vi "GUI.vi"() -> ()   [LabVIEW 2021]
uses:
  controls/ID Selector.ctl
  controls/UI Data.ctl
  controls/Data.ctl
  controls/ID.ctl
  controls/TCP states.ctl
  059b9806-6a42-4b51-9632-7dd4716d5fea.vi
  d48d9fbf-083e-4a49-8357-be6f50655bb8.vi
  d1c76d09-55ba-46af-828f-de7639a0dcdd.vi
  95893427-e2d0-46a1-b4a3-4e70b98dcc16.vi
  2dad5fc2-64a7-4bc6-978c-59d02dfdd1f4.vi
  2949da81-479a-477f-9d10-411d5337d71f.vi
  442cc11d-0c4b-4e6f-9aab-44bad20e65cf.vi
  aef3fa8d-d4ae-4391-a8c5-cd918d9f83e5.vi
  a61ae134-ce90-4c24-9a04-42d570ae496f.vi
  f3131f72-7d98-4291-8b40-3e2eb76ee77d.vi
  86390890-2633-40e9-acce-cca27de463dd.vi
  2bda4b71-a642-41ec-971a-aac1149cdb2e.vi
  4ba25f78-e02b-4593-a0a9-e7bfe2c227aa.vi
  b19a6172-c0db-45aa-bd96-f9eb8b4476d0.vi
  58187356-d8b0-41a2-b154-68928c7ad215.vi
  a77830ea-4afa-4eae-8504-e764fa7f6393.vi
  64a5f718-e64e-4ef8-854d-0519ac11c647.vi
  a36a24be-52b4-40ff-a07c-4f3c681fa51a.vi
  a822a74e-ca46-421e-8eac-677a4dba8bc9.vi
  651c30db-6f4a-4395-b9ba-95e4c80eae7c.vi
  ebd5c18a-2623-4cb2-8f61-688916ea3a38.vi
  3a8d74db-b308-4837-9c6e-c7dbc4062129.vi
  <vilib>/Utility/error.llb/Error Cluster From Error Code.vi
  styles/colors.vi
  <vilib>/ErrorRing/Error Ring.xnode
panel:
  out "ID:":string
  in  "Open part #":bool
  out "Parte number":string
  in  "Mode label":string="Mode:"
  in  "Options Button":bool
  in  "Mode:":T1
  in  "Start Button":bool
  out "Tab Control":enum32{"Micros", "Micro", "SSH"}(tab)
  in  "DH":bool
  in  "WH":bool
  in  "DA":bool
  in  "WM":bool
  in  "WA":bool
  in  "WC":bool
  in  "DS":bool
  in  "WS":bool
  in  "DM":bool
  in  "DC":bool
  in  "SM":bool
  in  "PWR":bool
  out "WS":string
  out "DS":string
  out "DM":string
  out "DC":string
  out "SM":string
  out "PWR":string
  out "WH":string
  out "DH":string
  out "DA":string
  out "WM":string
  out "WA":string
  out "WC":string
  out "Pass or fail":string
  out "Status":string caption="Conexión TCP-IP"
  out "version:":string
  in  "Save Button":bool
  in  "Path: 4.9.12.XXXX":path=path "C:/Users/ken_X/Documents/LabVIEW projects/Project-A/outset-medical/4.9.12.6034"
  in  "Path: Mi app":path=path "C:/Users/ken_X/Documents/LabVIEW projects/Project-A/outset-medical/Android OS"
  # "WS"
  # "DS"
  # "PWR"
  # "DM"
  # "SM"
  # "DC"
  # "WC"
  # "WH"
  # "DH"
  # "DA"
  # "WA"
  # "WM"
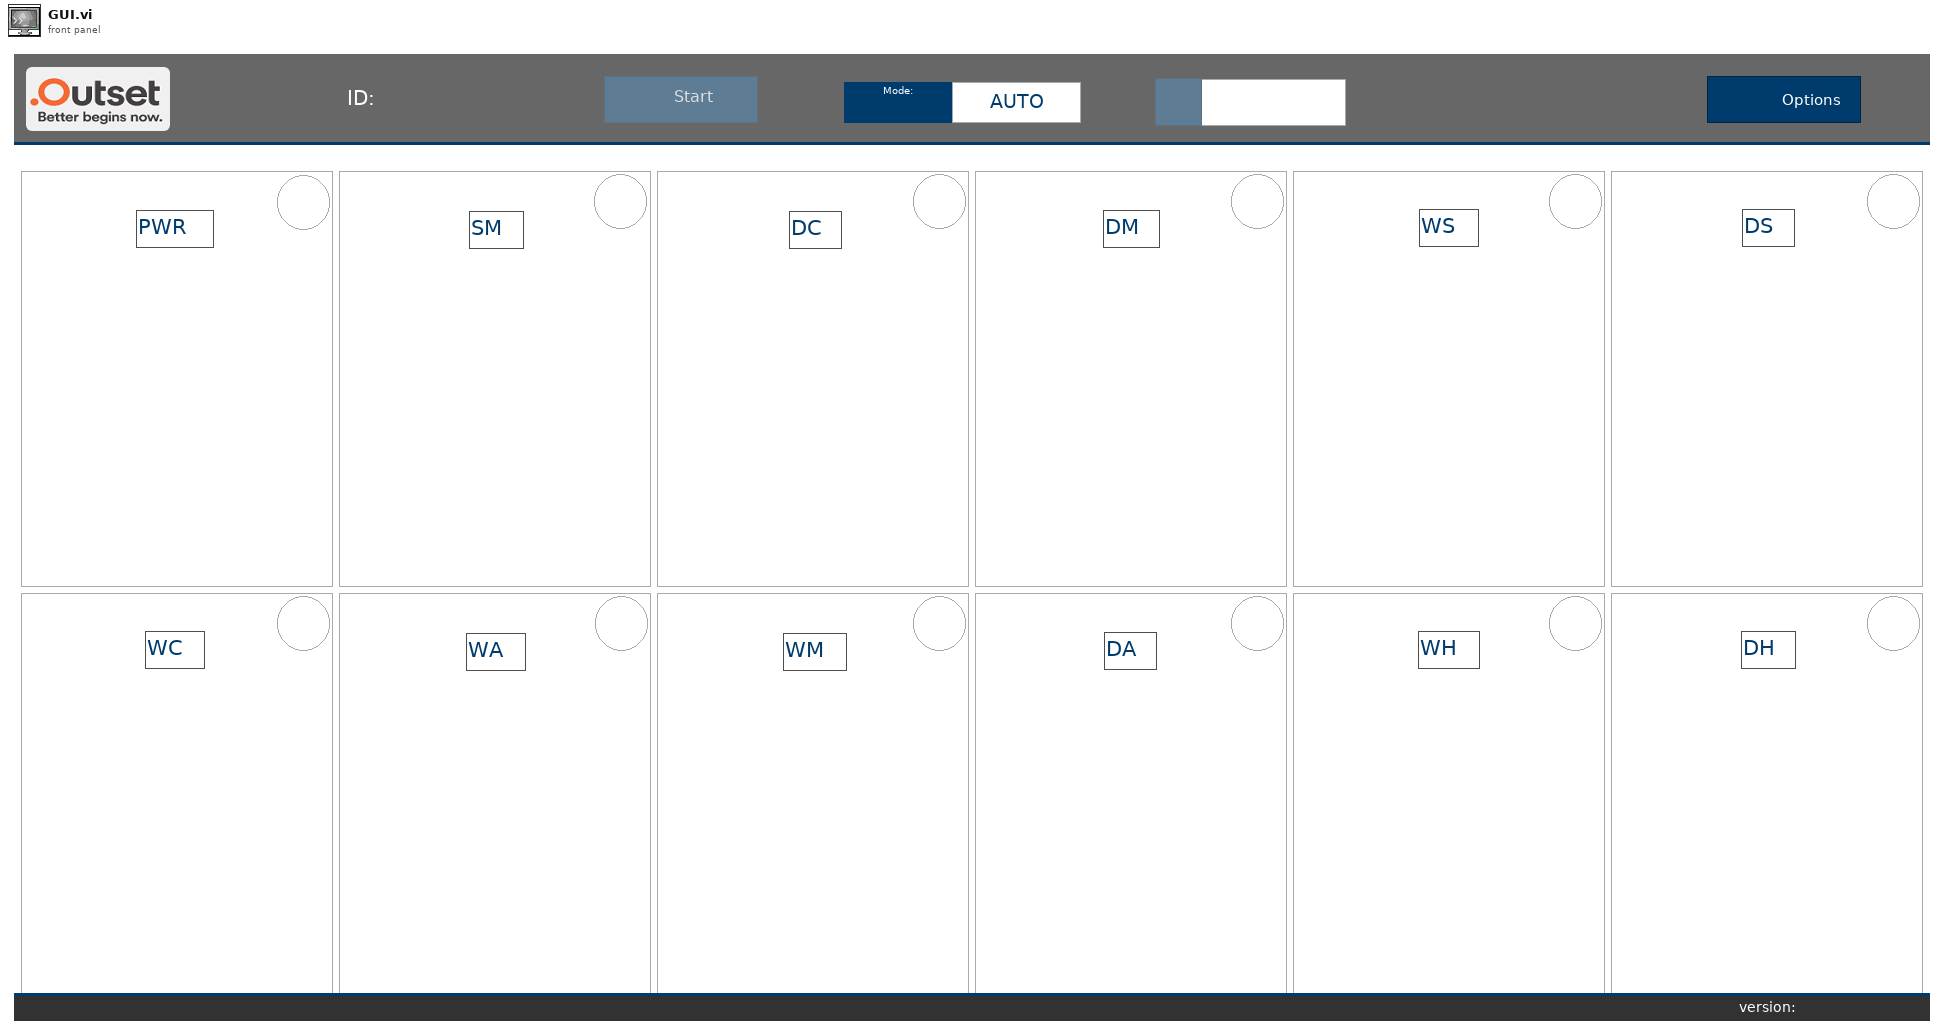
[diagram p1: front panel]
types:
  T1 = typedef "ID Selector.ctl" = enum16{"AUTO", "1 - PWR", "2 - SM", "3 - DC", "4 - DM", "5 - WS", "6 - DS", "7 - WC", "8 - WA", "9 - WM", "10 - DA", "11 - WH", "12 - DH"}
  T2 = enum8{"Enabled", "Disabled", "Disabled and Grayed Out"}
  T3 = typedef "Data.ctl" = cluster{"Path: 4.9.12.XXXX":path, "Path: Mi app":path, "Boolean refs":refnum<vi>[], "Indicator refs":refnum<vi>[], "USB left":u16, "Attemps left":u16, "Commands":string[], "ID":string, "Password":string, "Version":string, "Java":string, "URL":string, "DataProcessor?":string, "Pass?":string, "Checksum":string[]}
  T4 = typedef "UI Data.ctl" = cluster{"Path: Version":refnum<vi>, "Path: My app":refnum<vi>, "footer splitter":refnum<vi>, "Part number (.ini)":string}
  T5 = cluster{"primary color":u32, "secondary color":u32, "accent color":u32, "background color":u32, "accent s color":u32}
  T6 = cluster{"accent s color":u32, "accent s color":u32}
  T7 = typedef "ID.ctl" = enum16{"1 - PWR", "2 - SM", "3 - DC", "4 - DM", "5 - WS", "6 - DS", "7 - WC", "8 - WA", "9 - WM", "10 - DA", "11 - WH", "12 - DH"}
  T8 = typedef "TCP states.ctl" = string
  T9 = cluster{"Path: 4.9.12.XXXX":path, "Path: Mi app":path, "Username":string, "Password":string}
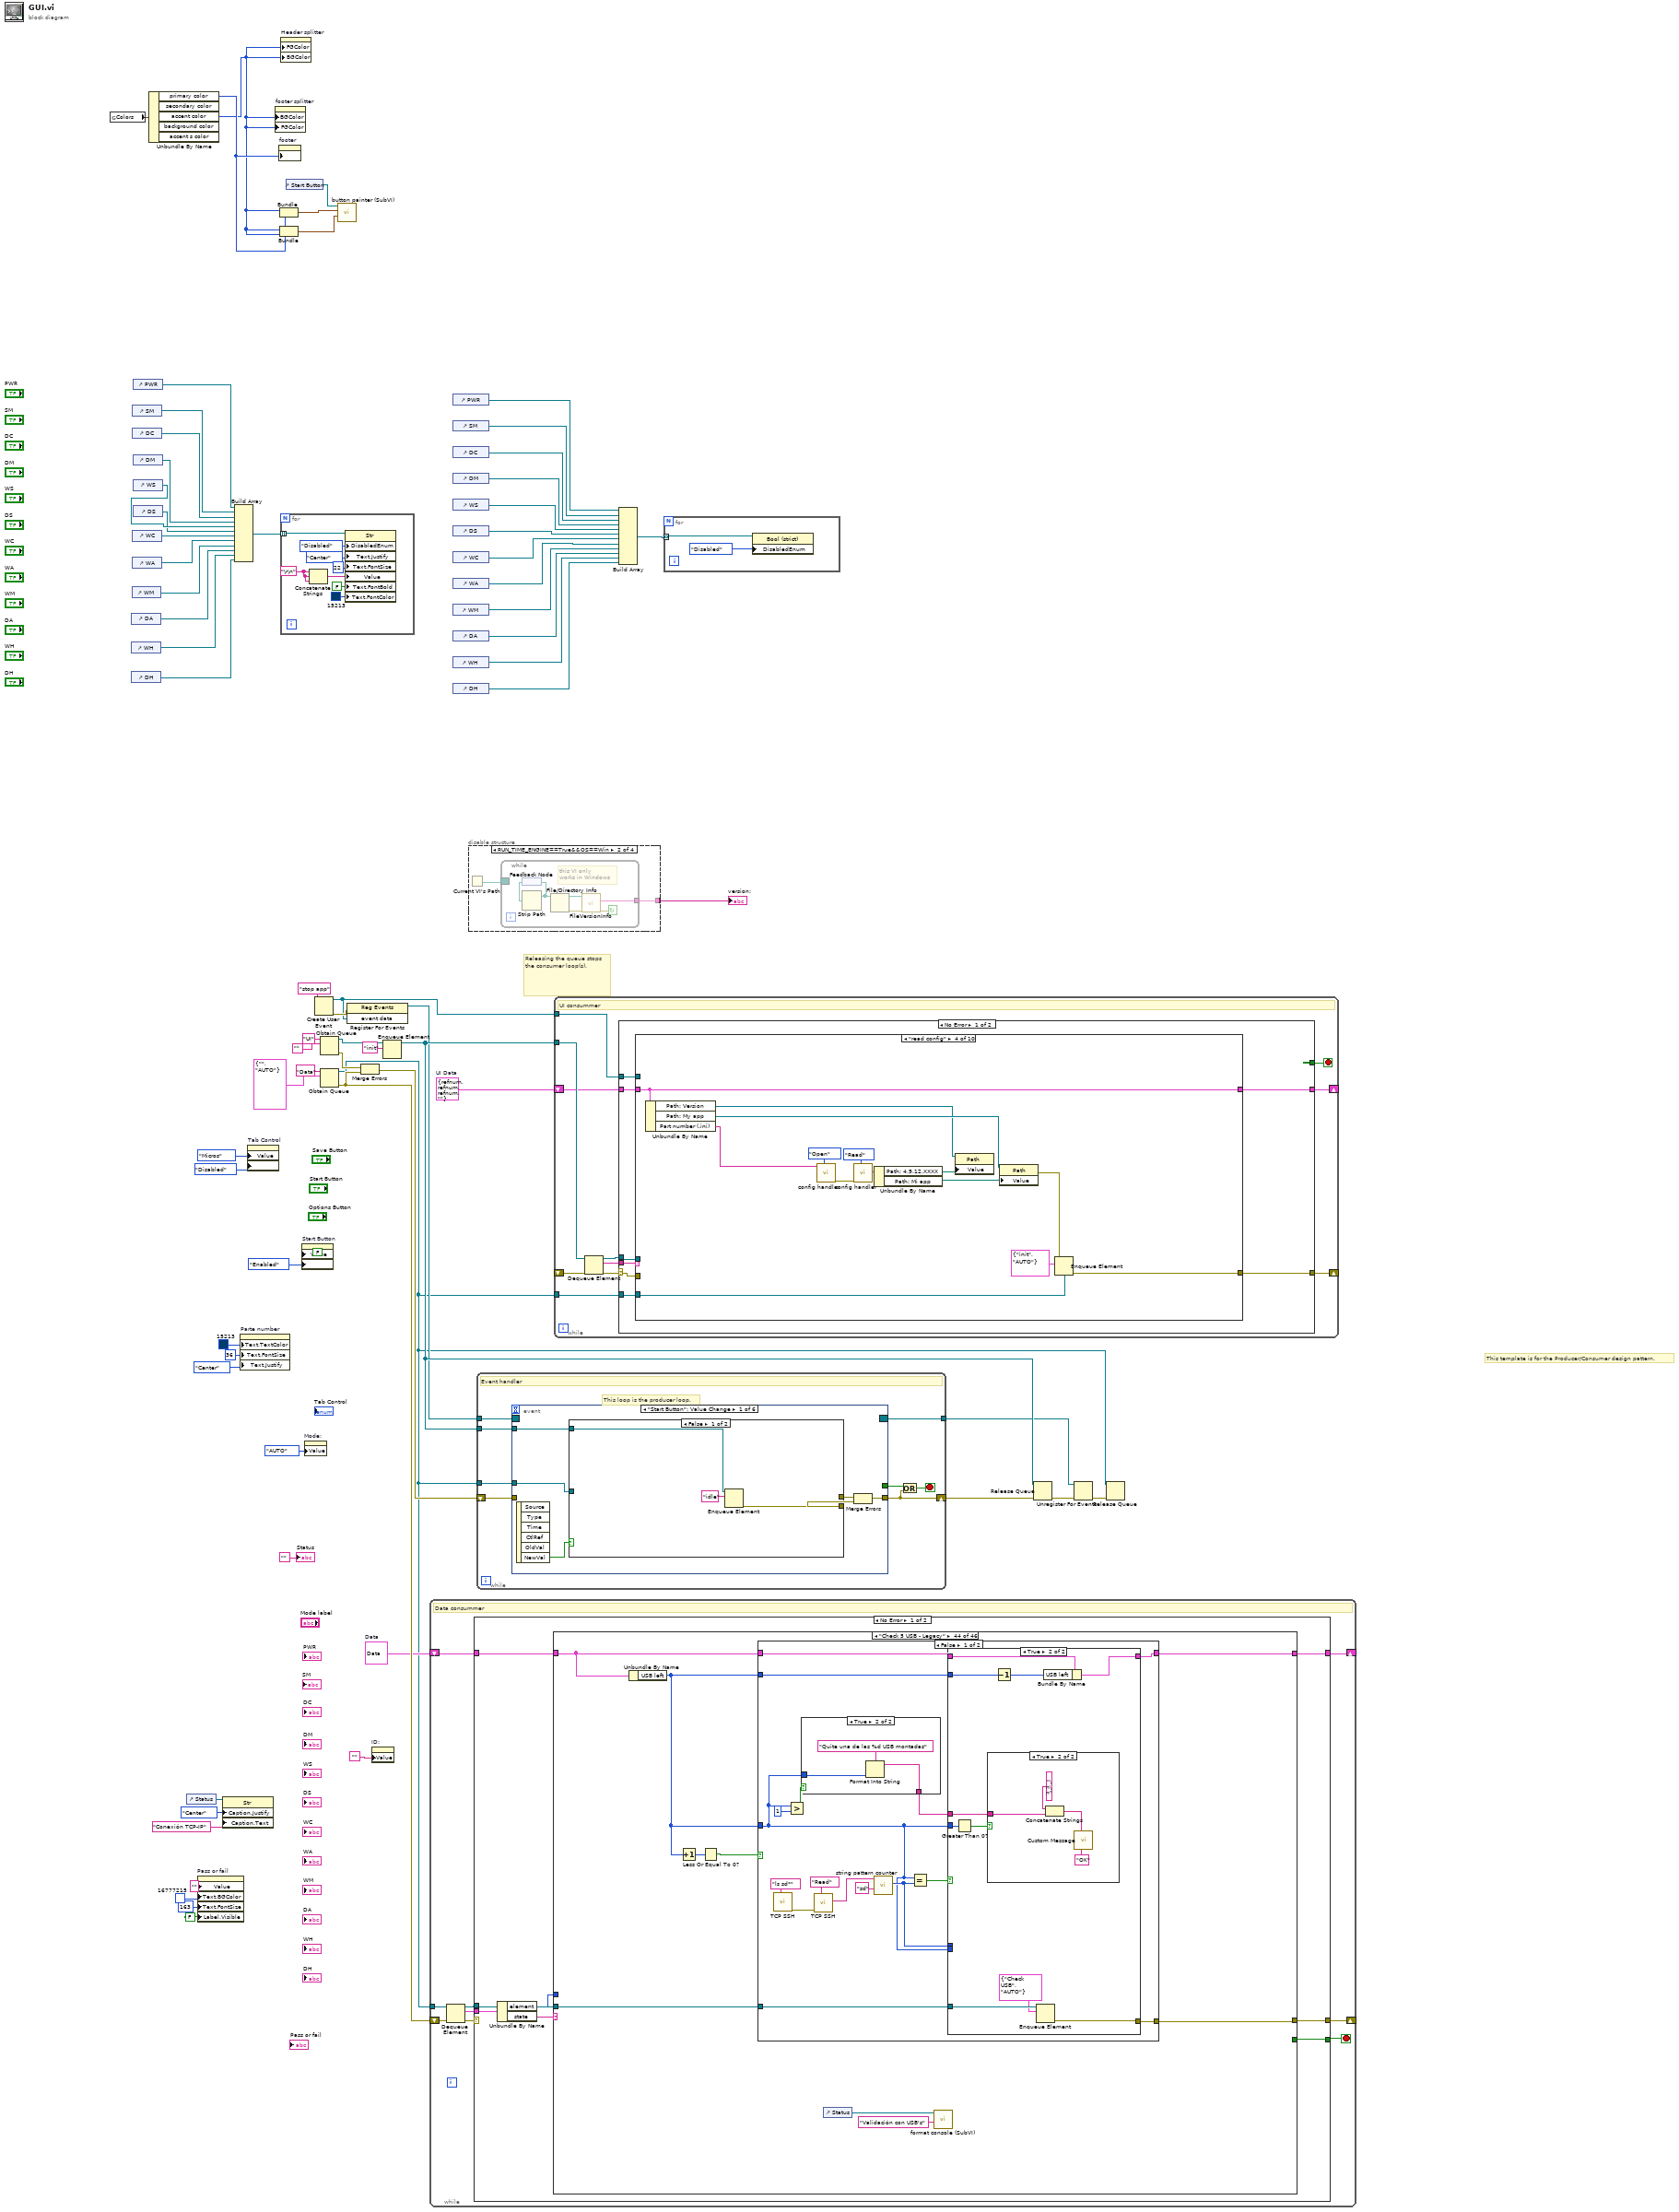
[diagram p0: block diagram]
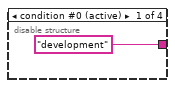
[diagram p2: hidden frame]
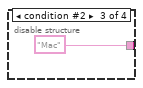
[diagram p3: hidden frame]
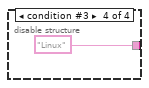
[diagram p4: hidden frame]
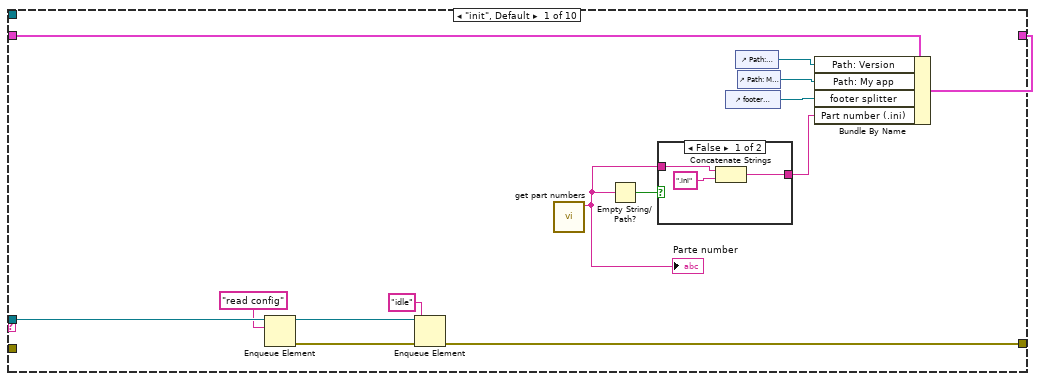
[diagram p5: hidden frame]
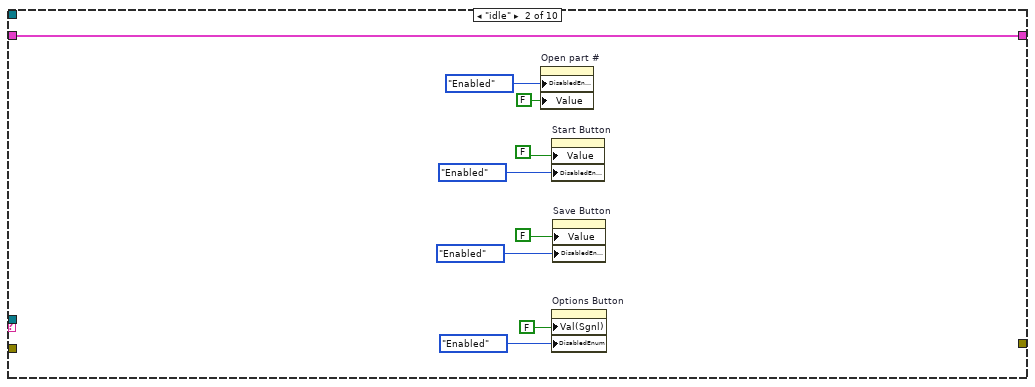
[diagram p7: hidden frame]
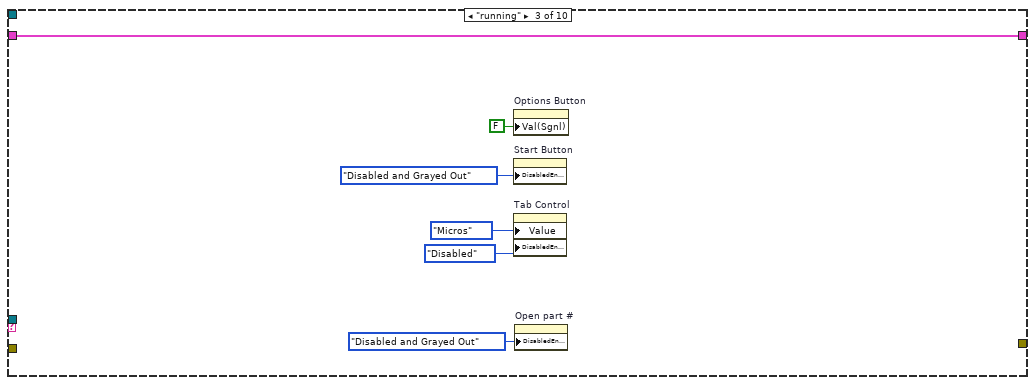
[diagram p8: hidden frame]
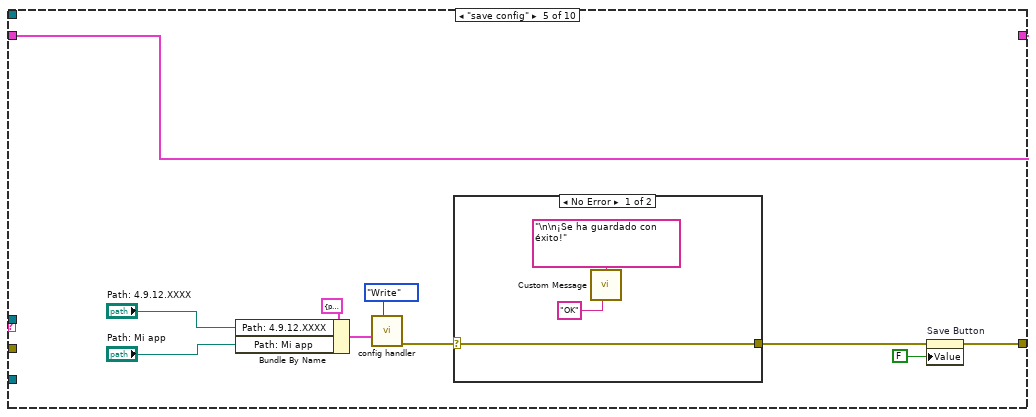
[diagram p9: hidden frame]
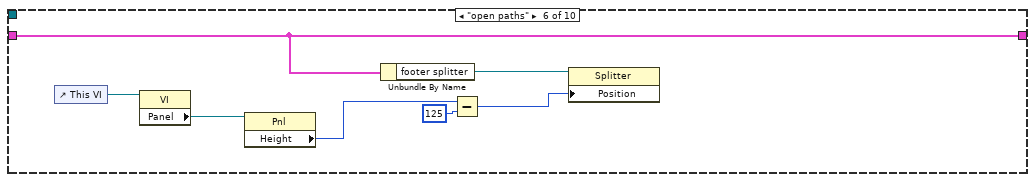
[diagram p11: hidden frame]
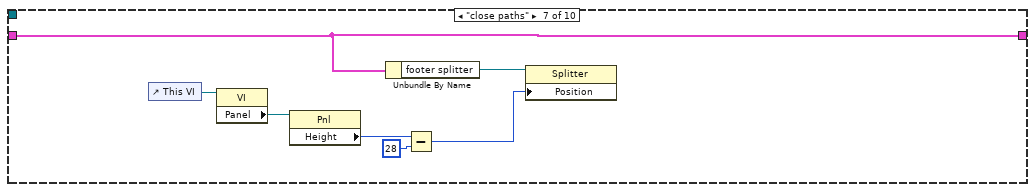
[diagram p12: hidden frame]
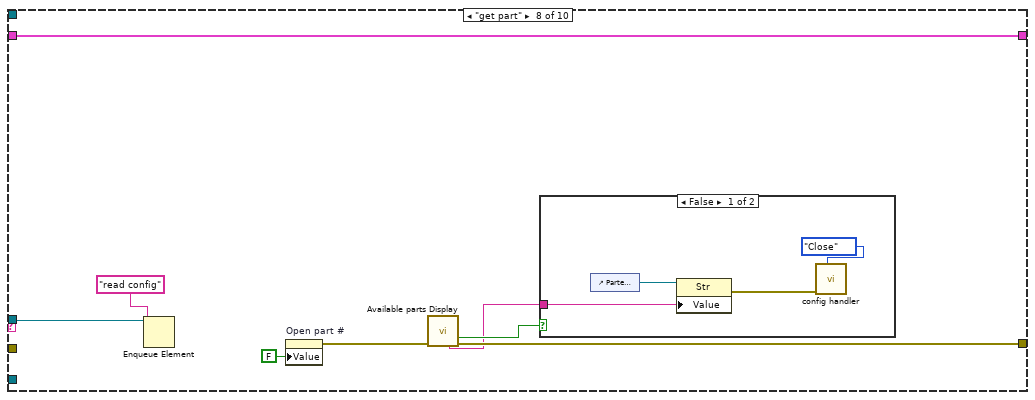
[diagram p13: hidden frame]
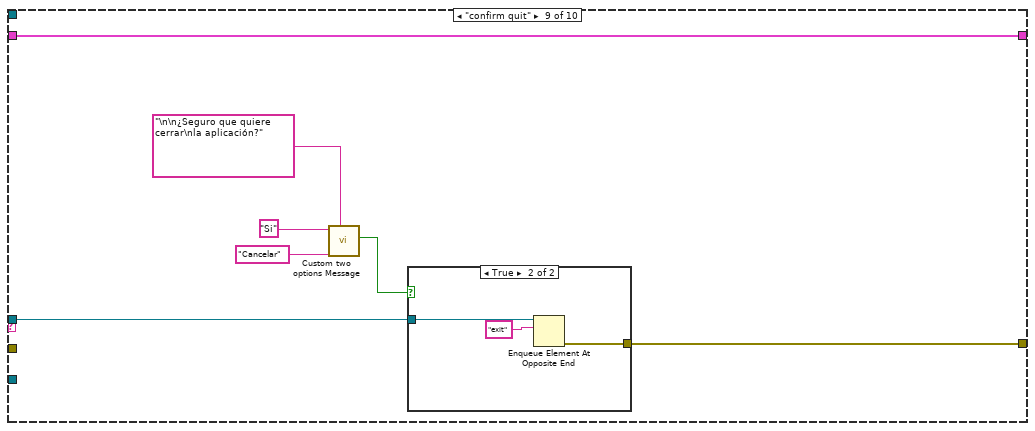
[diagram p15: hidden frame]
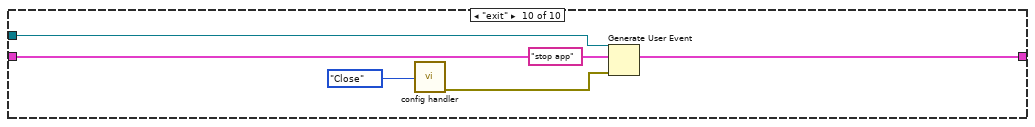
[diagram p17: hidden frame]
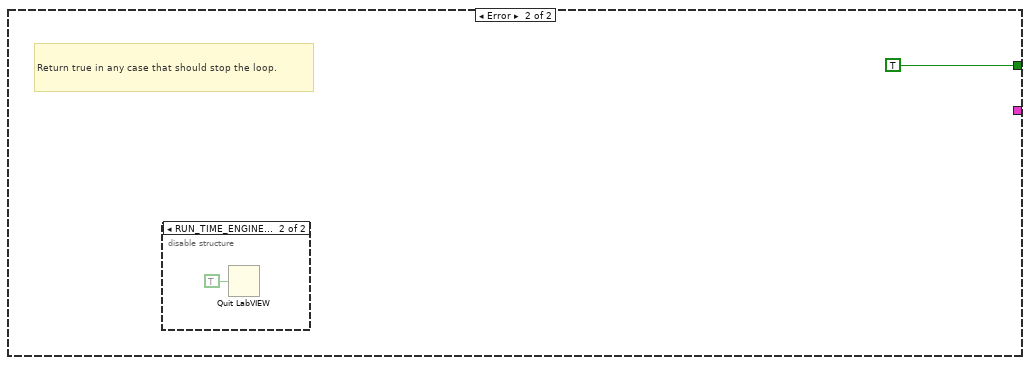
[diagram p18: hidden frame]
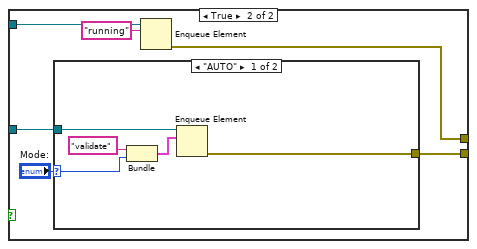
[diagram p20: hidden frame]
diagram:
  w27 = T3 {"Path: 4.9.12.XXXX"=path "", "Path: Mi app"=path "", "Boolean refs"=[], "Indicator refs"=[], "USB left"=0, "Attemps left"=0, "Commands"=[], "ID"="", "Password"="", "Version"="", "Java"="", "URL"="", "DataProcessor?"="", "Pass?"="", "Checksum"=[]}  # Data
  w37 = T4 {"Path: Version"=refnum, "Path: My app"=refnum, "footer splitter"=refnum, "Part number (.ini)"=""}  # UI Data
  # "Releasing the queue stops the consumer loop(s)."
  # "This template is for the Producer/Consumer design pattern."
  n1 = global read "colors.vi" "Colors"() -> (w71:T5)
  n2 = control-ref of="DA"() -> (w57:refnum<vi>)
  n3 = control-ref of="WH"() -> (w56:refnum<vi>)
  n4 = control-ref of="DH"() -> (w55:refnum<vi>)
  n5 = control-ref of="WM"() -> (w58:refnum<vi>)
  n6 = control-ref of="SM"() -> (w65:refnum<vi>)
  n7 = control-ref of="DC"() -> (w64:refnum<vi>)
  n8 = control-ref of="WC"() -> (w60:refnum<vi>)
  n9 = control-ref of="WA"() -> (w59:refnum<vi>)
  n10 = control-ref of="DM"() -> (w63:refnum<vi>)
  n11 = control-ref of="PWR"() -> (w66:refnum<vi>)
  n12 = control-ref of="WS"() -> (w62:refnum<vi>)
  n13 = control-ref of="DS"() -> (w61:refnum<vi>)
  n14 = Unbundle By Name(w71) -> ("primary color"=w68:u32, "accent color"=w67:u32)  [unwired: 3 out]
  n15 = control-ref of="Status"() -> (w12:refnum<vi>)
  n16 = property on="Pass or fail" class="Str"("Value"="" ("Pass or fail"), "Text.BGColor"=u32 16777215 ("Text.Text Colors:BG Color"), "Text.FontSize"=u32 163 ("Text.Font:Size"), "Label.Visible"=FALSE) -> ()  [unwired: 2 in, 2 out]
  n17 = property class="Str"(reference=w12, "Caption.Justify"=enum16{"Left", "Center", "Right"}."Center" ("Caption.Justification"), "Caption.Text"="Conexión TCP-IP") -> ()  [unwired: 1 in, 2 out]
  n18 = Build Array(w66, w65, w64, w63, w62, w61, w60, w59, w58, w57, w56, w55) -> (w54:refnum<vi>[])
  n19 = property on="Parte number" class="Str"("Text.TextColor"=u32 15213 ("Text.Text Colors:Text Color"), "Text.FontSize"=u32 36 ("Text.Font:Size"), "Text.Justify"=enum16{"Left", "Center", "Right"}."Center" ("Text.Justification")) -> ()  [unwired: 2 in, 2 out]
  n20 = property on="Tab Control" class="TabCtl (strict)"("Value"=enum32{"Micros", "Micro", "SSH"}."Micros" ("Tab Control"), "DisabledEnum"=T2."Disabled" ("Disabled")) -> ()  [unwired: 2 in, 2 out]
  n21 = property on="footer splitter" class="Splitter"("BGColor"=w67, "FGColor"=w67) -> ()  [unwired: 2 in, 2 out]
  n22 = property on="footer" class="Pane"("PaneColor"=w68) -> ()  [unwired: 2 in, 2 out]
  n23 = Bundle("accent color"=w67, "primary color"=w68) -> (w69:cluster{"accent color":u32, "primary color":u32})  [unwired: 1 in]
  n24 = Bundle("accent color"=w67, "accent color"=w67) -> (w70:cluster{"accent color":u32, "accent color":u32})  [unwired: 1 in]
  n25 = property on="Header splitter" class="Splitter"("FGColor"=w67, "BGColor"=w67) -> ()  [unwired: 2 in, 2 out]
  n26 = for {
    tunnel: w54 -> [w79] mode=indexing
    w74 = "\r\n"
    n27 = Concatenate Strings(w74, w74, w74) -> (w75:string)
    n28 = property on="Property Node" class="Str"(reference=w79, "DisabledEnum"=T2."Disabled" ("Disabled"), "Text.Justify"=enum16{"Left", "Center", "Right"}."Center" ("Text.Justification"), "Text.FontSize"=u32 22 ("Text.Font:Size"), "Value"=w75, "Text.FontBold"=FALSE ("Text.Font:Bold"), "Text.FontColor"=u32 15213 ("Text.Font:Color")) -> ()  [unwired: 1 in, 2 out]
  }
  n29 = control-ref of="Start Button"() -> (w19:refnum<vi>)
  n30 = property on="Start Button" class="Bool (strict)"("Value"=FALSE ("Save button"), "DisabledEnum"=T2."Enabled" ("Disabled")) -> ()  [unwired: 2 in, 2 out]
  n31 = property on="Mode:" class="Enum (strict)"("Value"=ID_Selector."AUTO" ("Mode:")) -> ()  [unwired: 2 in, 2 out]
  n32 = Create User Event(user event datatype="stop app" ("event data")) -> (user event=w35:refnum<user-event>, error out=w36:errorcluster)  [unwired: 1 in]
  n33 = Obtain Queue(name (unnamed)="UI", element data type="") -> (queue out=w39:refnum<queue>, error out=w31:errorcluster)  [unwired: 3 in, 1 out]
  n34 = Obtain Queue(name (unnamed)="Data", element data type=cluster{"state":string, "element":T1} {"state"="", "element"=enum."AUTO"}) -> (queue out=w17:refnum<queue>, error out=w28:errorcluster)  [unwired: 3 in, 1 out]
  n35 = call "button painter (SubVI).vi"("Off state"=w70, "On state"=w69, "Button ref in"=w19) -> ()  [unwired: 9 in]
  n36 = register-events(error in=w36, w35) -> (reference out=w34:refnum<event-registration>)  [unwired: 1 in, 1 out]
  n37 = Merge Errors(w31, w28) -> (w30:errorcluster)
  n38 = property on="ID:" class="Str"("Value"="") -> ()  [unwired: 2 in, 2 out]
  n39 = Enqueue Element(queue=w39, element="init") -> (queue out=w38:refnum<queue>)  [unwired: 2 in, 2 out]
  n40 = while {
    tunnel: w17 -> [w88]
    shift-right: [w82] -> _
    shift-left: w27 -> [w83]
    shift-right: [w81] -> _
    shift-left: w28 -> [w84]
    stop <- w80 stop-if-true
    # "Data consummer"
    n41 = Dequeue Element(queue=w88, error in (no error)=w84) -> (queue out=w85:refnum<queue>, element=w86:cluster{"state":string, "element":T1}, error out=w87:errorcluster)  [unwired: 1 in, 1 out]
    n42 = case shown="No Error" w87 {
      selector: w87 -> [_ w1380]
      tunnel: w86 -> [w96 _]
      tunnel: w85 -> [w93 w1392]
      tunnel: w83 -> [w92 w1368]
      tunnel: [w91 w1368] -> w82
      tunnel: [w94 w1386] -> w81
      tunnel: [w90 _] -> w80
      frame No Error {
        n43 = Unbundle By Name(w96) -> ("element"=w89:T1, "state"=w95:string)
        n44 = case shown="\"Check 5 USB - Legacy\"" w95 {
          tunnel: [_ _ w102 w123 _ w153 w180 w187 w230 w240 w264 w356 w451 w548 w735 _ _ w765 _ w801 w841 w847 w864 w881 w905 w925 w967 w990 w1008 w1038 w1048 w1069 w1085 w1096 w1100 w1118 w1139 w1161 w1178 w1202 w1229 w1240 w1254 w1282 w1347 w1364] -> w94
          tunnel: w93 -> [_ _ w101 _ _ w154 _ w188 w231 w241 w265 w355 w450 w547 w736 _ _ w766 _ w803 w842 w849 w863 w880 w906 w926 w951 w976 w1007 w1040 w1050 w1068 w1086 w1097 _ w1117 w1138 w1158 w1172 w1201 w1228 w1239 w1256 w1286 _ _]
          tunnel: w92 -> [w97 w98 w106 w128 w132 w159 w179 w186 w232 w237 w266 w279 w397 w577 w733 w749 w755 w759 w798 w800 w837 w843 w866 w883 w899 w927 w961 w992 w997 w1032 w1051 w1071 w1076 w1099 w1101 w1109 w1128 w1153 w1179 w1189 w1221 w1242 w1255 w1285 w1348 w1355]
          tunnel: [w97 w98 w106 w128 w132 w160 w178 w186 w233 w236 w266 w276 w395 w575 w732 w749 w754 w758 w798 w802 w837 w843 w866 w883 w899 w927 w961 w992 w996 w1032 w1051 w1071 w1076 w1099 w1101 w1112 w1127 w1153 w1179 w1196 w1220 w1242 w1255 w1284 w1348 w1355] -> w91
          tunnel: [_ TRUE ("Value (Signaling)") _ _ _ _ _ _ _ _ _ _ _ _ _ _ _ _ _ _ _ _ _ _ _ _ _ _ _ _ _ _ _ _ _ _ _ _ _ _ _ _ _ _ _ _] -> w90
          tunnel: w89 -> [_ _ w100 w121 _ _ _ _ _ _ _ _ _ _ _ _ _ _ _ _ _ _ _ _ _ _ _ _ _ _ _ _ _ _ _ _ _ _ _ _ _ _ _ _ _ _]
          frame "idle", Default {
          }
          frame "kill loop" {
          }
          frame "validate 4.9.12" {
            n45 = Unbundle By Name(w106) -> ("Path: 4.9.12.XXXX"=w105:path)
            n46 = call <vilib>:"Check if File or Folder Exists.vi"("path"=w105) -> ("file or folder exists?"=w104:bool)  [unwired: 8 in, 2 out]
            n47 = case shown="False" w104 {
              selector: w104 -> [_ w116]
              tunnel: [_ w116] -> w103
              frame False {
                n48 = call "Custom Error Message.vi"("MSG"="\nNo existe la carpeta 4.9.12.XXXX \nen la ruta configurada") -> ()  [unwired: 11 in]
              }
              frame True {
              }
            }
            n49 = case shown="True" w103 {
              tunnel: [w109 w114] -> w102
              tunnel: w101 -> [w108 w113]
              tunnel: w100 -> [_ w112]
              frame False {
                n50 = Enqueue Element(queue=w108, element=cluster{"state":string, "element":T1} {"state"="idle", "element"=enum."AUTO"}) -> (error out=w109:errorcluster)  [unwired: 2 in, 2 out]
              }
              frame True {
                n51 = Bundle("program one", "element"=w112) -> (w110:cluster{string, "element":T1})  [unwired: 1 in]
                n52 = Enqueue Element(queue=w113, element=w110) -> (error out=w114:errorcluster)  [unwired: 2 in, 2 out]
              }
            }
          }
          frame "program one" {
            n53 = Unbundle By Name(w128) -> ("Indicator refs"=w120:refnum<vi>[], "Commands"=w122:string[], "Boolean refs"=w117:refnum<vi>[], "Path: 4.9.12.XXXX"=w130:path)
            n54 = call "To ID (SubVI).vi"("element"=w121) -> ("ID"=w129:T7)  [unwired: 10 in]
            n55 = call "Clear leds (SubVI).vi"("Boolean refs"=w117) -> ("Boolean refs out"=w118:refnum<vi>[])  [unwired: 10 in]
            n56 = call "Clear screens (SubVI).vi"("String refs"=w120) -> ("String refs out"=w119:refnum<vi>[])  [unwired: 10 in]
            n57 = Index Array(array=w119, index=w129) -> (element=w127:refnum<vi>)
            n58 = call "Programer.vi"("ID"=w129, "version path"=w130, "Boolean refs"=w118, "Commands"=w122) -> ("error out"=w124:errorcluster, "Response"=w126:string)  [unwired: 4 in, 2 out]
            n59 = call "Concatenate by ref (SubVI).vi"("Response"=w126, "String ref in"=w127) -> ()  [unwired: 9 in, 1 out]
            n60 = property on="Start Button" class="Bool (strict)"(error in=w124, "Val(Sgnl)"=FALSE ("Start Button")) -> (error out=w123:errorcluster)  [unwired: 1 in, 1 out]
          }
          frame "clear screens" {
            n61 = Unbundle By Name(w132) -> ("Indicator refs"=w131:refnum<vi>[])
            n62 = for {
              tunnel: w131 -> [w135] mode=indexing
              w134 = "\r\n"
              n63 = Concatenate Strings(w134, w134, w134) -> (w133:string)
              n64 = property on="Property Node" class="Str"(reference=w135, "Value"=w133) -> ()  [unwired: 1 in, 2 out]
            }
          }
          frame "init" {
            n65 = control-ref of="PWR"() -> (w172:refnum<vi>)
            n66 = control-ref of="SM"() -> (w171:refnum<vi>)
            n67 = control-ref of="DC"() -> (w170:refnum<vi>)
            n68 = control-ref of="DM"() -> (w169:refnum<vi>)
            n69 = control-ref of="WS"() -> (w168:refnum<vi>)
            n70 = control-ref of="DS"() -> (w167:refnum<vi>)
            n71 = control-ref of="WC"() -> (w166:refnum<vi>)
            n72 = control-ref of="WA"() -> (w165:refnum<vi>)
            n73 = control-ref of="WM"() -> (w164:refnum<vi>)
            n74 = control-ref of="DA"() -> (w163:refnum<vi>)
            n75 = control-ref of="WH"() -> (w162:refnum<vi>)
            n76 = control-ref of="DH"() -> (w161:refnum<vi>)
            n77 = Build Array(w172, w171, w170, w169, w168, w167, w166, w165, w164, w163, w162, w161) -> (w151:refnum<vi>[])
            n78 = for {
              tunnel: w151 -> [w175] mode=indexing
              n79 = property class="Bool (strict)"(reference=w175, "Value"=FALSE) -> ()  [unwired: 1 in, 2 out]
              n80 = call "button painter (SubVI).vi"("Off state"=cluster{"accent color":u32, "accent color":u32} {"accent color"=16777216, "accent color"=16777216}, "On state"=T6 {"accent s color"=16711680, "accent s color"=16711680}, "Button ref in"=w175) -> ()  [unwired: 9 in]
            }
            n81 = control-ref of="DA"() -> (w141:refnum<vi>)
            n82 = control-ref of="WH"() -> (w140:refnum<vi>)
            n83 = control-ref of="DH"() -> (w139:refnum<vi>)
            n84 = control-ref of="WM"() -> (w142:refnum<vi>)
            n85 = control-ref of="SM"() -> (w149:refnum<vi>)
            n86 = control-ref of="DC"() -> (w148:refnum<vi>)
            n87 = control-ref of="WC"() -> (w144:refnum<vi>)
            n88 = control-ref of="WA"() -> (w143:refnum<vi>)
            n89 = control-ref of="DM"() -> (w147:refnum<vi>)
            n90 = control-ref of="PWR"() -> (w150:refnum<vi>)
            n91 = control-ref of="WS"() -> (w146:refnum<vi>)
            n92 = control-ref of="DS"() -> (w145:refnum<vi>)
            n93 = Enqueue Element(queue=w154, element=cluster{"state":string, "element":T1} {"state"="commands", "element"=enum."AUTO"}) -> (error out=w153:errorcluster)  [unwired: 2 in, 2 out]
            n94 = call "config handler.vi"("Operation"=enum16{"Open", "Write", "Read", "Close"}."Read") -> ("Read values"=w157:T9)  [unwired: 9 in, 1 out]
            n95 = Unbundle By Name(w157) -> ("Password"=w136:string, "Path: 4.9.12.XXXX"=w156:path, "Path: Mi app"=w155:path)
            n96 = Build Array(w150, w149, w148, w147, w146, w145, w144, w143, w142, w141, w140, w139) -> (w138:refnum<vi>[])
            n97 = Bundle By Name(cluster=w159, "Password"=w136, "Path: 4.9.12.XXXX"=w156, "Path: Mi app"=w155, "Boolean refs"=w151, "Indicator refs"=w138, "Attemps left"=u16 2 ("Racks left")) -> (w160:T3)
          }
          frame "commands" {
            n98 = call "Command builder.vi"() -> ("error out"=w180:errorcluster, "Commands"=w177:string[])  [unwired: 10 in]
            n99 = Bundle By Name(cluster=w179, "Commands"=w177) -> (w178:T3)
          }
          frame "validate" {
            n100 = Unbundle By Name(w186) -> ("Path: 4.9.12.XXXX"=w194:path, "Path: Mi app"=w195:path)
            n101 = disable-structure "Conditional Disable Structure" shown="RUN_TIME_ENGINE==True&&OS==Win" {
              disable-tunnel: [w202 w203] -> w181
              frame condition #0 (active) {
                w201 = "C:\\temp\\plink.exe "  # Script File Name
                n102 = String To Path(string=w201) -> (path=w202:path)
              }
              frame condition #1 {
                w205 = "data\\plink.exe"  # Script File Name
                n103 = call <vilib>:"Application Directory.vi"() -> ("Application Directory"=w204:path)
                n104 = Build Path(base path=w204, name or relative path=w205) -> (appended path=w203:path)
              }
            }
            n105 = call <vilib>:"Check if File or Folder Exists.vi"("path"=path "C:/Python27") -> ("file or folder exists?"=w197:bool)  [unwired: 8 in, 2 out]
            n106 = call <vilib>:"Check if File or Folder Exists.vi"("path"=w195) -> ("file or folder exists?"=w192:bool)  [unwired: 8 in, 2 out]
            n107 = case shown="False" w197 {
              selector: w197 -> [_ w221]
              tunnel: [_ w221] -> w196
              frame False {
                n108 = call "Custom Error Message.vi"("MSG"="No se tiene la versión correcta de Python, \no la versión actual esta corrompida.") -> ()  [unwired: 11 in]
              }
              frame True {
              }
            }
            n109 = call <vilib>:"Check if File or Folder Exists.vi"("path"=w194) -> ("file or folder exists?"=w193:bool)  [unwired: 8 in, 2 out]
            n110 = case shown="False" w193 {
              selector: w193 -> [_ w219]
              tunnel: [_ w219] -> w190
              frame False {
                n111 = call "Custom Error Message.vi"("MSG"="\nNo existe la carpeta 4.9.12.XXXX \nen la ruta configurada") -> ()  [unwired: 11 in]
              }
              frame True {
              }
            }
            n112 = case shown="False" w192 {
              selector: w192 -> [_ w217]
              tunnel: [_ w217] -> w191
              frame False {
                n113 = call "Custom Error Message.vi"("MSG"="\nNo existe la carpeta \"Mi app\"\nen la ruta configurada") -> ()  [unwired: 11 in]
              }
              frame True {
              }
            }
            n114 = call <vilib>:"Check if File or Folder Exists.vi"("path"=w181) -> ("file or folder exists?"=w182:bool)  [unwired: 8 in, 2 out]
            n115 = case shown="False" w182 {
              selector: w182 -> [_ w200]
              tunnel: [_ w200] -> w183
              frame False {
                n116 = call "Custom Error Message.vi"("MSG"="El programa \"plink.exe\" no se encuentra \nen la ruta: C:\\Cardcage\\data\\plink.exe\n") -> ()  [unwired: 11 in]
              }
              frame True {
              }
            }
            n117 = Compound Arithmetic op=AND(w190, w191, w196, w183) -> (w189:bool)
            n118 = case shown="True" w189 {
              tunnel: w188 -> [_ w209]
              tunnel: [w206 w208] -> w187
              frame False {
                n119 = property on="Start Button" class="Bool (strict)"("Value"=TRUE) -> (error out=w206:errorcluster)  [unwired: 2 in, 1 out]
              }
              frame True {
                n120 = disable-structure shown="Enabled" {
                  disable-tunnel: w209 -> [w211 w215]
                  disable-tunnel: [w212 w214] -> w208
                  frame Enabled {
                    n121 = Enqueue Element(queue=w211, element=cluster{"state":string, "element":T1} {"state"="scan id", "element"=enum."AUTO"}) -> (error out=w212:errorcluster)  [unwired: 2 in, 2 out]
                  }
                  frame Disabled {
                    n122 = Enqueue Element(queue=w215, element=cluster{"state":string, "element":T1} {"state"="Ping", "element"=enum."AUTO"}) -> (error out=w214:errorcluster)  [unwired: 2 in, 2 out]
                  }
                }
              }
            }
            n123 = Unbundle By Name(w186) -> ("Boolean refs"=w185:refnum<vi>[], "Indicator refs"=w184:refnum<vi>[])  [unwired: 1 out]
            n124 = call "Clear screens (SubVI).vi"("String refs"=w184) -> ()  [unwired: 10 in, 1 out]
            n125 = call "Clear leds (SubVI).vi"("Boolean refs"=w185) -> ()  [unwired: 10 in, 1 out]
          }
          frame "scan id" {
            n126 = property on="Parte number" class="Str"() -> ("Value"=w228:string)  [unwired: 2 in, 2 out]
            n127 = Enqueue Element(queue=w231, element=cluster{"state":string, "element":T1} {"state"="pwr", "element"=enum."AUTO"}) -> (error out=w230:errorcluster)  [unwired: 2 in, 2 out]
            n128 = call "Scan id.vi"() -> ("out"=w222:string)  [unwired: 10 in, 1 out]
            "ID:" <- w222
            n129 = Bundle By Name(cluster=w232, "ID"=w222, "Version"=w228, "Java"="", "URL"="", "DataProcessor?"="False", "Pass?"="False", "Checksum"=string[] []) -> (w233:T3)
          }
          frame "pwr" {
            w243 = ID."1 - PWR" ("ID")
            n130 = Unbundle By Name(w237) -> ("Indicator refs"=w238:refnum<vi>[], "Commands"=w244:string[], "Boolean refs"=w248:refnum<vi>[], "Path: 4.9.12.XXXX"=w247:path)
            n131 = call "Clear screens (SubVI).vi"("String refs"=w238) -> ("String refs out"=w239:refnum<vi>[])  [unwired: 10 in]
            n132 = Index Array(array=w239, index=w243) -> (element=w246:refnum<vi>)
            n133 = call "Programer.vi"("ID"=w243, "version path"=w247, "Boolean refs"=w248, "Commands"=w244) -> ("error?"=w242:bool, "Checksum"=w235:string, "Response"=w245:string)  [unwired: 4 in, 1 out]
            n134 = call "Concatenate by ref (SubVI).vi"("Response"=w245, "String ref in"=w246) -> ()  [unwired: 9 in, 1 out]
            n135 = case shown="True" w242 {
              tunnel: w241 -> [w250 w254]
              tunnel: [w251 w253] -> w240
              frame False {
                n136 = Enqueue Element(queue=w250, element=cluster{"state":string, "element":T1} {"state"="SPS", "element"=enum."AUTO"}) -> (error out=w251:errorcluster)  [unwired: 2 in, 2 out]
              }
              frame True {
                n137 = call "Custom two options Message.vi"("MSG"="\nHubo un error al programar PWR. \nAsegurece que la maquina esta prendida, y\nque todo este bien conectado.\n", "Red text"="Abortar", "Green text"="Reintentar") -> ("Ok?"=w252:bool)  [unwired: 8 in]
                n138 = case shown="True" w252 {
                  tunnel: w254 -> [_ w262]
                  tunnel: [w258 w260] -> w253
                  frame False {
                    n139 = xnode "Error Ring"() -> ("error out"=w258:errorcluster)
                  }
                  frame True {
                    n140 = Enqueue Element(queue=w262, element=cluster{"state":string, "element":T1} {"state"="pwr", "element"=enum."AUTO"}) -> (error out=w260:errorcluster)  [unwired: 2 in, 2 out]
                  }
                }
              }
            }
            n141 = Build Array(w235) -> (w234:string[])
            n142 = Bundle By Name(cluster=w237, "Checksum"=w234) -> (w236:T3)
          }
          frame "SPS" {
            n143 = flat-sequence {
              tunnel: w265 -> [w269]
              tunnel: [w269] -> w263
              tunnel: [w271] -> w264
              tunnel: w263 -> [w273]
              frame #0 {
                n144 = call "Custom Message.vi"("Boolean Text"="¡SPS Presionado!", "MSG"="\nPresione el botón SPS para energizar toda la maquina" ("message")) -> ()  [unwired: 10 in]
              }
              frame #1 {
                n145 = Enqueue Element(queue=w273, element=cluster{"state":string, "element":T1} {"state"="program all", "element"=enum."AUTO"}) -> (error out=w274:errorcluster)  [unwired: 2 in, 2 out]
                n146 = call "Stall Data Flow.vim"("value in"=w274, "milliseconds to wait"=u32 5000) -> ("value out"=w271:errorcluster)  [unwired: 1 out]
              }
            }
          }
          frame "program all" {
            n147 = Unbundle By Name(w279) -> ("Indicator refs"=w354:refnum<vi>[], "Path: 4.9.12.XXXX"=w335:path, "Boolean refs"=w336:refnum<vi>[], "Commands"=w337:string[])
            n148 = call "Stall Data Flow.vim"("value in"=w337, "milliseconds to wait"=u32 1) -> ("value out"=w305:string[])  [unwired: 1 out]
            n149 = call "Stall Data Flow.vim"("value in"=w337, "milliseconds to wait"=u32 100) -> ("value out"=w301:string[])  [unwired: 1 out]
            n150 = call "Stall Data Flow.vim"("value in"=w337, "milliseconds to wait"=u32 625) -> ("value out"=w297:string[])  [unwired: 1 out]
            n151 = call "Stall Data Flow.vim"("value in"=w337, "milliseconds to wait"=u32 300) -> ("value out"=w303:string[])  [unwired: 1 out]
            n152 = call "Stall Data Flow.vim"("value in"=w337, "milliseconds to wait"=u32 300) -> ("value out"=w299:string[])  [unwired: 1 out]
            n153 = call "Stall Data Flow.vim"("value in"=w337, "milliseconds to wait"=u32 750) -> ("value out"=w307:string[])  [unwired: 1 out]
            n154 = call "Stall Data Flow.vim"("value in"=w337, "milliseconds to wait"=u32 100) -> ("value out"=w309:string[])  [unwired: 1 out]
            n155 = call "Stall Data Flow.vim"("value in"=w337, "milliseconds to wait"=u32 500) -> ("value out"=w360:string[])  [unwired: 1 out]
            n156 = call "Stall Data Flow.vim"("value in"=w337, "milliseconds to wait"=u32 150) -> ("value out"=w358:string[])  [unwired: 1 out]
            n157 = call "Stall Data Flow.vim"("value in"=w337, "milliseconds to wait"=u32 1) -> ("value out"=w295:string[])  [unwired: 1 out]
            n158 = call "Programer.vi"("ID"=ID."2 - SM", "version path"=w335, "Boolean refs"=w336, "Commands"=w360) -> ("error?"=w319:bool, "Checksum"=w290:string, "Response"=w353:string)  [unwired: 4 in, 1 out]
            n159 = call "Programer.vi"("ID"=ID."3 - DC", "version path"=w335, "Boolean refs"=w336, "Commands"=w358) -> ("error?"=w318:bool, "Checksum"=w289:string, "Response"=w350:string)  [unwired: 4 in, 1 out]
            n160 = call "Programer.vi"("ID"=ID."4 - DM", "version path"=w335, "Boolean refs"=w336, "Commands"=w337) -> ("error?"=w317:bool, "Checksum"=w288:string, "Response"=w348:string)  [unwired: 4 in, 1 out]
            n161 = call "Programer.vi"("ID"=ID."5 - WS", "version path"=w335, "Boolean refs"=w336, "Commands"=w309) -> ("error?"=w316:bool, "Checksum"=w287:string, "Response"=w346:string)  [unwired: 4 in, 1 out]
            n162 = call "Programer.vi"("ID"=ID."6 - DS", "version path"=w335, "Boolean refs"=w336, "Commands"=w307) -> ("error?"=w315:bool, "Checksum"=w286:string, "Response"=w345:string)  [unwired: 4 in, 1 out]
            n163 = call "Programer.vi"("ID"=ID."7 - WC", "version path"=w335, "Boolean refs"=w336, "Commands"=w297) -> ("error?"=w312:bool, "Checksum"=w285:string, "Response"=w344:string)  [unwired: 4 in, 1 out]
            n164 = call "Programer.vi"("ID"=ID."8 - WA", "version path"=w335, "Boolean refs"=w336, "Commands"=w305) -> ("error?"=w311:bool, "Checksum"=w284:string, "Response"=w343:string)  [unwired: 4 in, 1 out]
            n165 = call "Programer.vi"("ID"=ID."9 - WM", "version path"=w335, "Boolean refs"=w336, "Commands"=w303) -> ("error?"=w310:bool, "Checksum"=w283:string, "Response"=w342:string)  [unwired: 4 in, 1 out]
            n166 = call "Programer.vi"("ID"=ID."10 - DA", "version path"=w335, "Boolean refs"=w336, "Commands"=w299) -> ("error?"=w293:bool, "Checksum"=w282:string, "Response"=w334:string)  [unwired: 4 in, 1 out]
            n167 = call "Programer.vi"("ID"=ID."11 - WH", "version path"=w335, "Boolean refs"=w336, "Commands"=w301) -> ("error?"=w292:bool, "Checksum"=w281:string, "Response"=w333:string)  [unwired: 4 in, 1 out]
            n168 = call "Programer.vi"("ID"=ID."12 - DH", "version path"=w335, "Boolean refs"=w336, "Commands"=w295) -> ("error?"=w291:bool, "Checksum"=w280:string, "Response"=w330:string)  [unwired: 4 in, 1 out]
            n169 = Index Array(array=w354) -> (element #2=w352:refnum<vi>, element #3=w351:refnum<vi>, element #4=w349:refnum<vi>, element #5=w347:refnum<vi>, element #6=w341:refnum<vi>, element #7=w340:refnum<vi>, element #8=w339:refnum<vi>, element #9=w338:refnum<vi>, element #10=w332:refnum<vi>, element #11=w331:refnum<vi>, element #12=w329:refnum<vi>)  [unwired: 12 in, 1 out]
            n170 = call "Concatenate by ref (SubVI).vi"("Response"=w342, "String ref in"=w338) -> ()  [unwired: 9 in, 1 out]
            n171 = call "Concatenate by ref (SubVI).vi"("Response"=w334, "String ref in"=w332) -> ()  [unwired: 9 in, 1 out]
            n172 = call "Concatenate by ref (SubVI).vi"("Response"=w353, "String ref in"=w352) -> ()  [unwired: 9 in, 1 out]
            n173 = call "Concatenate by ref (SubVI).vi"("Response"=w348, "String ref in"=w349) -> ()  [unwired: 9 in, 1 out]
            n174 = call "Concatenate by ref (SubVI).vi"("Response"=w346, "String ref in"=w347) -> ()  [unwired: 9 in, 1 out]
            n175 = call "Concatenate by ref (SubVI).vi"("Response"=w345, "String ref in"=w341) -> ()  [unwired: 9 in, 1 out]
            n176 = call "Concatenate by ref (SubVI).vi"("Response"=w344, "String ref in"=w340) -> ()  [unwired: 9 in, 1 out]
            n177 = call "Concatenate by ref (SubVI).vi"("Response"=w343, "String ref in"=w339) -> ()  [unwired: 9 in, 1 out]
            n178 = call "Concatenate by ref (SubVI).vi"("Response"=w333, "String ref in"=w331) -> ()  [unwired: 9 in, 1 out]
            n179 = call "Concatenate by ref (SubVI).vi"("Response"=w330, "String ref in"=w329) -> ()  [unwired: 9 in, 1 out]
            n180 = call "Concatenate by ref (SubVI).vi"("Response"=w350, "String ref in"=w351) -> ()  [unwired: 9 in, 1 out]
            n181 = Build Array(w319, w318, w317, w316, w315, w312, w311, w310, w293, w292, w291) -> (w314:bool[])
            n182 = Unbundle By Name(w279) -> ("Checksum"=w278:string[])
            n183 = Or Array Elements(Boolean array=w314) -> (logical OR=w313:bool)
            n184 = case shown="True" w313 {
              tunnel: [w364 w367] -> w356
              tunnel: w355 -> [w363 w368]
              frame False {
                n185 = Enqueue Element(queue=w363, element=cluster{"state":string, "element":T1} {"state"="Validate USB", "element"=enum."AUTO"}) -> (error out=w364:errorcluster)  [unwired: 2 in, 2 out]
              }
              frame True {
                n186 = Enqueue Element(queue=w368, element=cluster{"state":string, "element":T1} {"state"="reprogram", "element"=enum."AUTO"}) -> (error out=w367:errorcluster)  [unwired: 2 in, 2 out]
              }
            }
            n187 = Build Array(w290, w289, w288, w287, w286, w285, w284, w283, w282, w281, w280) -> (w277:string[])
            n188 = Build Array (concatenate)(w278, w277) -> (w275:string[])
            n189 = Bundle By Name(cluster=w279, "Checksum"=w275) -> (w276:T3)
          }
          frame "reprogram" {
            n190 = Unbundle By Name(w397) -> ("Indicator refs"=w405:refnum<vi>[], "Commands"=w417:string[], "Boolean refs"=w416:refnum<vi>[], "Path: 4.9.12.XXXX"=w415:path, "Checksum"=w392:string[])
            n191 = Index Array(array=w392, index #1=1 ("index")) -> (element #1=w379:string, element #2=w378:string, element #3=w377:string, element #4=w376:string, element #5=w375:string, element #6=w374:string, element #7=w373:string, element #8=w372:string, element #9=w371:string, element #10=w370:string, element #11=w369:string)  [unwired: 10 in]
            n192 = call "ref to boolean.vi"("Boolean refs"=w416) -> ("Boolean values"=w420:bool[])  [unwired: 9 in, 1 out]
            n193 = Index Array(array=w420) -> (element #2=w419:bool, element #3=w418:bool, element #4=w414:bool, element #5=w413:bool, element #6=w412:bool, element #7=w411:bool, element #8=w410:bool, element #9=w409:bool, element #10=w408:bool, element #11=w407:bool, element #12=w406:bool)  [unwired: 12 in, 1 out]
            n194 = call "Clear screens (SubVI).vi"("String refs"=w405) -> ("String refs out"=w404:refnum<vi>[])  [unwired: 10 in]
            n195 = case shown="False" w419 {
              tunnel: [_ w538] -> w449
              tunnel: [_ w537] -> w427
              tunnel: w415 -> [_ w536]
              tunnel: w416 -> [_ w535]
              tunnel: w417 -> [_ w534]
              tunnel: [w532 w533] -> w390
              tunnel: w379 -> [w532 _]
              frame False {
              }
              frame True {
                n196 = call "Programer.vi"("ID"=ID."2 - SM", "version path"=w536, "Boolean refs"=w535, "Commands"=w534) -> ("error?"=w537:bool, "Checksum"=w533:string, "Response"=w538:string)  [unwired: 4 in, 1 out]
              }
            }
            n197 = case shown="False" w418 {
              tunnel: [_ w530] -> w446
              tunnel: [_ w529] -> w426
              tunnel: w417 -> [_ w528]
              tunnel: w416 -> [_ w527]
              tunnel: w415 -> [_ w526]
              tunnel: [w524 w525] -> w389
              tunnel: w378 -> [w524 _]
              frame False {
              }
              frame True {
                n198 = call "Programer.vi"("ID"=ID."3 - DC", "version path"=w526, "Boolean refs"=w527, "Commands"=w528) -> ("error?"=w529:bool, "Checksum"=w525:string, "Response"=w530:string)  [unwired: 4 in, 1 out]
              }
            }
            n199 = case shown="False" w414 {
              tunnel: [_ w523] -> w444
              tunnel: [_ w521] -> w425
              tunnel: w417 -> [_ w520]
              tunnel: w416 -> [_ w519]
              tunnel: w415 -> [_ w518]
              tunnel: [w516 w517] -> w388
              tunnel: w377 -> [w516 _]
              frame False {
              }
              frame True {
                n200 = call "Programer.vi"("ID"=ID."4 - DM", "version path"=w518, "Boolean refs"=w519, "Commands"=w520) -> ("error?"=w521:bool, "Checksum"=w517:string, "Response"=w523:string)  [unwired: 4 in, 1 out]
              }
            }
            n201 = case shown="False" w413 {
              tunnel: [_ w511] -> w442
              tunnel: [_ w514] -> w424
              tunnel: w416 -> [_ w513]
              tunnel: w415 -> [_ w512]
              tunnel: w417 -> [_ w510]
              tunnel: [w508 w509] -> w387
              tunnel: w376 -> [w508 _]
              frame False {
              }
              frame True {
                n202 = call "Programer.vi"("ID"=ID."5 - WS", "version path"=w512, "Boolean refs"=w513, "Commands"=w510) -> ("error?"=w514:bool, "Checksum"=w509:string, "Response"=w511:string)  [unwired: 4 in, 1 out]
              }
            }
            n203 = case shown="False" w412 {
              tunnel: [_ w507] -> w441
              tunnel: [_ w505] -> w423
              tunnel: w417 -> [_ w504]
              tunnel: w416 -> [_ w503]
              tunnel: w415 -> [_ w502]
              tunnel: [w500 w501] -> w386
              tunnel: w375 -> [w500 _]
              frame False {
              }
              frame True {
                n204 = call "Programer.vi"("ID"=ID."6 - DS", "version path"=w502, "Boolean refs"=w503, "Commands"=w504) -> ("error?"=w505:bool, "Checksum"=w501:string, "Response"=w507:string)  [unwired: 4 in, 1 out]
              }
            }
            n205 = case shown="False" w411 {
              tunnel: [_ w499] -> w440
              tunnel: [_ w497] -> w403
              tunnel: w417 -> [_ w496]
              tunnel: w416 -> [_ w495]
              tunnel: w415 -> [_ w494]
              tunnel: [w492 w493] -> w385
              tunnel: w374 -> [w492 _]
              frame False {
              }
              frame True {
                n206 = call "Programer.vi"("ID"=ID."7 - WC", "version path"=w494, "Boolean refs"=w495, "Commands"=w496) -> ("error?"=w497:bool, "Checksum"=w493:string, "Response"=w499:string)  [unwired: 4 in, 1 out]
              }
            }
            n207 = case shown="False" w410 {
              tunnel: [_ w491] -> w439
              tunnel: [_ w489] -> w402
              tunnel: w417 -> [_ w488]
              tunnel: w416 -> [_ w487]
              tunnel: w415 -> [_ w486]
              tunnel: [w484 w485] -> w384
              tunnel: w373 -> [w484 _]
              frame False {
              }
              frame True {
                n208 = call "Programer.vi"("ID"=ID."8 - WA", "version path"=w486, "Boolean refs"=w487, "Commands"=w488) -> ("error?"=w489:bool, "Checksum"=w485:string, "Response"=w491:string)  [unwired: 4 in, 1 out]
              }
            }
            n209 = case shown="False" w409 {
              tunnel: [_ w483] -> w438
              tunnel: [_ w481] -> w401
              tunnel: w417 -> [_ w480]
              tunnel: w416 -> [_ w479]
              tunnel: w415 -> [_ w478]
              tunnel: [w476 w477] -> w383
              tunnel: w372 -> [w476 _]
              frame False {
              }
              frame True {
                n210 = call "Programer.vi"("ID"=ID."9 - WM", "version path"=w478, "Boolean refs"=w479, "Commands"=w480) -> ("error?"=w481:bool, "Checksum"=w477:string, "Response"=w483:string)  [unwired: 4 in, 1 out]
              }
            }
            n211 = case shown="False" w408 {
              tunnel: [_ w475] -> w433
              tunnel: [_ w473] -> w400
              tunnel: w417 -> [_ w472]
              tunnel: w416 -> [_ w471]
              tunnel: w415 -> [_ w470]
              tunnel: [w468 w469] -> w382
              tunnel: w371 -> [w468 _]
              frame False {
              }
              frame True {
                n212 = call "Programer.vi"("ID"=ID."10 - DA", "version path"=w470, "Boolean refs"=w471, "Commands"=w472) -> ("error?"=w473:bool, "Checksum"=w469:string, "Response"=w475:string)  [unwired: 4 in, 1 out]
              }
            }
            n213 = case shown="False" w407 {
              tunnel: [_ w467] -> w432
              tunnel: [_ w465] -> w399
              tunnel: w417 -> [_ w464]
              tunnel: w416 -> [_ w463]
              tunnel: w415 -> [_ w462]
              tunnel: [w460 w461] -> w381
              tunnel: w370 -> [w460 _]
              frame False {
              }
              frame True {
                n214 = call "Programer.vi"("ID"=ID."11 - WH", "version path"=w462, "Boolean refs"=w463, "Commands"=w464) -> ("error?"=w465:bool, "Checksum"=w461:string, "Response"=w467:string)  [unwired: 4 in, 1 out]
              }
            }
            n215 = case shown="False" w406 {
              tunnel: [_ w459] -> w429
              tunnel: [_ w457] -> w398
              tunnel: w417 -> [_ w456]
              tunnel: w416 -> [_ w455]
              tunnel: w415 -> [_ w454]
              tunnel: [w452 w453] -> w380
              tunnel: w369 -> [w452 _]
              frame False {
              }
              frame True {
                n216 = call "Programer.vi"("ID"=ID."12 - DH", "version path"=w454, "Boolean refs"=w455, "Commands"=w456) -> ("error?"=w457:bool, "Checksum"=w453:string, "Response"=w459:string)  [unwired: 4 in, 1 out]
              }
            }
            n217 = Index Array(array=w404) -> (element #2=w448:refnum<vi>, element #3=w447:refnum<vi>, element #4=w445:refnum<vi>, element #5=w443:refnum<vi>, element #6=w437:refnum<vi>, element #7=w436:refnum<vi>, element #8=w435:refnum<vi>, element #9=w434:refnum<vi>, element #10=w431:refnum<vi>, element #11=w430:refnum<vi>, element #12=w428:refnum<vi>)  [unwired: 12 in, 1 out]
            n218 = call "Concatenate by ref (SubVI).vi"("Response"=w438, "String ref in"=w434) -> ()  [unwired: 9 in, 1 out]
            n219 = call "Concatenate by ref (SubVI).vi"("Response"=w433, "String ref in"=w431) -> ()  [unwired: 9 in, 1 out]
            n220 = call "Concatenate by ref (SubVI).vi"("Response"=w449, "String ref in"=w448) -> ()  [unwired: 9 in, 1 out]
            n221 = call "Concatenate by ref (SubVI).vi"("Response"=w444, "String ref in"=w445) -> ()  [unwired: 9 in, 1 out]
            n222 = call "Concatenate by ref (SubVI).vi"("Response"=w442, "String ref in"=w443) -> ()  [unwired: 9 in, 1 out]
            n223 = call "Concatenate by ref (SubVI).vi"("Response"=w441, "String ref in"=w437) -> ()  [unwired: 9 in, 1 out]
            n224 = call "Concatenate by ref (SubVI).vi"("Response"=w440, "String ref in"=w436) -> ()  [unwired: 9 in, 1 out]
            n225 = call "Concatenate by ref (SubVI).vi"("Response"=w439, "String ref in"=w435) -> ()  [unwired: 9 in, 1 out]
            n226 = call "Concatenate by ref (SubVI).vi"("Response"=w432, "String ref in"=w430) -> ()  [unwired: 9 in, 1 out]
            n227 = call "Concatenate by ref (SubVI).vi"("Response"=w429, "String ref in"=w428) -> ()  [unwired: 9 in, 1 out]
            n228 = call "Concatenate by ref (SubVI).vi"("Response"=w446, "String ref in"=w447) -> ()  [unwired: 9 in, 1 out]
            n229 = Unbundle By Name(w397) -> ("Checksum"=w396:string[])
            n230 = Build Array(w427, w426, w425, w424, w423, w403, w402, w401, w400, w399, w398) -> (w422:bool[])
            n231 = Or Array Elements(Boolean array=w422) -> (logical OR=w421:bool)
            n232 = case shown="True" w421 {
              tunnel: [w542 w545] -> w451
              tunnel: w450 -> [w541 w544]
              frame False {
                n233 = Enqueue Element(queue=w541, element=cluster{"state":string, "element":T1} {"state"="Validate USB", "element"=enum."AUTO"}) -> (error out=w542:errorcluster)  [unwired: 2 in, 2 out]
              }
              frame True {
                n234 = Enqueue Element(queue=w544, element=cluster{"state":string, "element":T1} {"state"="reprogram 2", "element"=enum."AUTO"}) -> (error out=w545:errorcluster)  [unwired: 2 in, 2 out]
              }
            }
            n235 = Replace Array Subset(array=w396, new element #1=w390, index #1=1 ("index"), new element #2=w389, new element #3=w388, new element #4=w387, new element #5=w386, new element #6=w385, new element #7=w384, new element #8=w383, new element #9=w382, new element #10=w381, new element #11=w380) -> (w394:string[])  [unwired: 10 in]
            n236 = Bundle By Name(cluster=w397, "Checksum"=w394) -> (w395:T3)
          }
          frame "reprogram 2" {
            n237 = Unbundle By Name(w577) -> ("Indicator refs"=w585:refnum<vi>[], "Commands"=w597:string[], "Boolean refs"=w596:refnum<vi>[], "Path: 4.9.12.XXXX"=w595:path, "Checksum"=w572:string[])
            n238 = Index Array(array=w572, index #1=1 ("index")) -> (element #1=w559:string, element #2=w558:string, element #3=w557:string, element #4=w556:string, element #5=w555:string, element #6=w554:string, element #7=w553:string, element #8=w552:string, element #9=w551:string, element #10=w550:string, element #11=w549:string)  [unwired: 10 in]
            n239 = call "ref to boolean.vi"("Boolean refs"=w596) -> ("Boolean values"=w600:bool[])  [unwired: 9 in, 1 out]
            n240 = Index Array(array=w600) -> (element #2=w599:bool, element #3=w598:bool, element #4=w594:bool, element #5=w593:bool, element #6=w592:bool, element #7=w591:bool, element #8=w590:bool, element #9=w589:bool, element #10=w588:bool, element #11=w587:bool, element #12=w586:bool)  [unwired: 12 in, 1 out]
            n241 = call "Clear screens (SubVI).vi"("String refs"=w585) -> ("String refs out"=w584:refnum<vi>[])  [unwired: 10 in]
            n242 = case shown="False" w599 {
              tunnel: [_ w729] -> w628
              tunnel: [_ w728] -> w606
              tunnel: w595 -> [_ w727]
              tunnel: w596 -> [_ w726]
              tunnel: w597 -> [_ w725]
              tunnel: [w723 w724] -> w570
              tunnel: w559 -> [w723 _]
              frame False {
              }
              frame True {
                n243 = call "Programer.vi"("ID"=ID."2 - SM", "version path"=w727, "Boolean refs"=w726, "Commands"=w725) -> ("error?"=w728:bool, "Checksum"=w724:string, "Response"=w729:string)  [unwired: 4 in, 1 out]
              }
            }
            n244 = case shown="False" w598 {
              tunnel: [_ w721] -> w625
              tunnel: [_ w720] -> w605
              tunnel: w597 -> [_ w719]
              tunnel: w596 -> [_ w718]
              tunnel: w595 -> [_ w717]
              tunnel: [w715 w716] -> w569
              tunnel: w558 -> [w715 _]
              frame False {
              }
              frame True {
                n245 = call "Programer.vi"("ID"=ID."3 - DC", "version path"=w717, "Boolean refs"=w718, "Commands"=w719) -> ("error?"=w720:bool, "Checksum"=w716:string, "Response"=w721:string)  [unwired: 4 in, 1 out]
              }
            }
            n246 = case shown="False" w594 {
              tunnel: [_ w714] -> w623
              tunnel: [_ w712] -> w604
              tunnel: w597 -> [_ w711]
              tunnel: w596 -> [_ w710]
              tunnel: w595 -> [_ w709]
              tunnel: [w707 w708] -> w568
              tunnel: w557 -> [w707 _]
              frame False {
              }
              frame True {
                n247 = call "Programer.vi"("ID"=ID."4 - DM", "version path"=w709, "Boolean refs"=w710, "Commands"=w711) -> ("error?"=w712:bool, "Checksum"=w708:string, "Response"=w714:string)  [unwired: 4 in, 1 out]
              }
            }
            n248 = case shown="False" w593 {
              tunnel: [_ w702] -> w621
              tunnel: [_ w705] -> w603
              tunnel: w596 -> [_ w704]
              tunnel: w595 -> [_ w703]
              tunnel: w597 -> [_ w701]
              tunnel: [w699 w700] -> w567
              tunnel: w556 -> [w699 _]
              frame False {
              }
              frame True {
                n249 = call "Programer.vi"("ID"=ID."5 - WS", "version path"=w703, "Boolean refs"=w704, "Commands"=w701) -> ("error?"=w705:bool, "Checksum"=w700:string, "Response"=w702:string)  [unwired: 4 in, 1 out]
              }
            }
            n250 = case shown="False" w592 {
              tunnel: [_ w698] -> w620
              tunnel: [_ w696] -> w602
              tunnel: w597 -> [_ w695]
              tunnel: w596 -> [_ w694]
              tunnel: w595 -> [_ w693]
              tunnel: [w691 w692] -> w566
              tunnel: w555 -> [w691 _]
              frame False {
              }
              frame True {
                n251 = call "Programer.vi"("ID"=ID."6 - DS", "version path"=w693, "Boolean refs"=w694, "Commands"=w695) -> ("error?"=w696:bool, "Checksum"=w692:string, "Response"=w698:string)  [unwired: 4 in, 1 out]
              }
            }
            n252 = case shown="False" w591 {
              tunnel: [_ w690] -> w619
              tunnel: [_ w688] -> w583
              tunnel: w597 -> [_ w687]
              tunnel: w596 -> [_ w686]
              tunnel: w595 -> [_ w685]
              tunnel: [w683 w684] -> w565
              tunnel: w554 -> [w683 _]
              frame False {
              }
              frame True {
                n253 = call "Programer.vi"("ID"=ID."7 - WC", "version path"=w685, "Boolean refs"=w686, "Commands"=w687) -> ("error?"=w688:bool, "Checksum"=w684:string, "Response"=w690:string)  [unwired: 4 in, 1 out]
              }
            }
            n254 = case shown="False" w590 {
              tunnel: [_ w682] -> w618
              tunnel: [_ w680] -> w582
              tunnel: w597 -> [_ w679]
              tunnel: w596 -> [_ w678]
              tunnel: w595 -> [_ w677]
              tunnel: [w675 w676] -> w564
              tunnel: w553 -> [w675 _]
              frame False {
              }
              frame True {
                n255 = call "Programer.vi"("ID"=ID."8 - WA", "version path"=w677, "Boolean refs"=w678, "Commands"=w679) -> ("error?"=w680:bool, "Checksum"=w676:string, "Response"=w682:string)  [unwired: 4 in, 1 out]
              }
            }
            n256 = case shown="False" w589 {
              tunnel: [_ w674] -> w617
              tunnel: [_ w672] -> w581
              tunnel: w597 -> [_ w671]
              tunnel: w596 -> [_ w670]
              tunnel: w595 -> [_ w669]
              tunnel: [w667 w668] -> w563
              tunnel: w552 -> [w667 _]
              frame False {
              }
              frame True {
                n257 = call "Programer.vi"("ID"=ID."9 - WM", "version path"=w669, "Boolean refs"=w670, "Commands"=w671) -> ("error?"=w672:bool, "Checksum"=w668:string, "Response"=w674:string)  [unwired: 4 in, 1 out]
              }
            }
            n258 = case shown="False" w588 {
              tunnel: [_ w666] -> w612
              tunnel: [_ w664] -> w580
              tunnel: w597 -> [_ w663]
              tunnel: w596 -> [_ w662]
              tunnel: w595 -> [_ w661]
              tunnel: [w659 w660] -> w562
              tunnel: w551 -> [w659 _]
              frame False {
              }
              frame True {
                n259 = call "Programer.vi"("ID"=ID."10 - DA", "version path"=w661, "Boolean refs"=w662, "Commands"=w663) -> ("error?"=w664:bool, "Checksum"=w660:string, "Response"=w666:string)  [unwired: 4 in, 1 out]
              }
            }
            n260 = case shown="False" w587 {
              tunnel: [_ w658] -> w611
              tunnel: [_ w656] -> w579
              tunnel: w597 -> [_ w655]
              tunnel: w596 -> [_ w654]
              tunnel: w595 -> [_ w653]
              tunnel: [w651 w652] -> w561
              tunnel: w550 -> [w651 _]
              frame False {
              }
              frame True {
                n261 = call "Programer.vi"("ID"=ID."11 - WH", "version path"=w653, "Boolean refs"=w654, "Commands"=w655) -> ("error?"=w656:bool, "Checksum"=w652:string, "Response"=w658:string)  [unwired: 4 in, 1 out]
              }
            }
            n262 = case shown="False" w586 {
              tunnel: [_ w650] -> w608
              tunnel: [_ w648] -> w578
              tunnel: w597 -> [_ w647]
              tunnel: w596 -> [_ w646]
              tunnel: w595 -> [_ w645]
              tunnel: [w643 w644] -> w560
              tunnel: w549 -> [w643 _]
              frame False {
              }
              frame True {
                n263 = call "Programer.vi"("ID"=ID."12 - DH", "version path"=w645, "Boolean refs"=w646, "Commands"=w647) -> ("error?"=w648:bool, "Checksum"=w644:string, "Response"=w650:string)  [unwired: 4 in, 1 out]
              }
            }
            n264 = Index Array(array=w584) -> (element #2=w627:refnum<vi>, element #3=w626:refnum<vi>, element #4=w624:refnum<vi>, element #5=w622:refnum<vi>, element #6=w616:refnum<vi>, element #7=w615:refnum<vi>, element #8=w614:refnum<vi>, element #9=w613:refnum<vi>, element #10=w610:refnum<vi>, element #11=w609:refnum<vi>, element #12=w607:refnum<vi>)  [unwired: 12 in, 1 out]
            n265 = call "Concatenate by ref (SubVI).vi"("Response"=w617, "String ref in"=w613) -> ()  [unwired: 9 in, 1 out]
            n266 = call "Concatenate by ref (SubVI).vi"("Response"=w612, "String ref in"=w610) -> ()  [unwired: 9 in, 1 out]
            n267 = call "Concatenate by ref (SubVI).vi"("Response"=w628, "String ref in"=w627) -> ()  [unwired: 9 in, 1 out]
            n268 = call "Concatenate by ref (SubVI).vi"("Response"=w623, "String ref in"=w624) -> ()  [unwired: 9 in, 1 out]
            n269 = call "Concatenate by ref (SubVI).vi"("Response"=w621, "String ref in"=w622) -> ()  [unwired: 9 in, 1 out]
            n270 = call "Concatenate by ref (SubVI).vi"("Response"=w620, "String ref in"=w616) -> ()  [unwired: 9 in, 1 out]
            n271 = call "Concatenate by ref (SubVI).vi"("Response"=w619, "String ref in"=w615) -> ()  [unwired: 9 in, 1 out]
            n272 = call "Concatenate by ref (SubVI).vi"("Response"=w618, "String ref in"=w614) -> ()  [unwired: 9 in, 1 out]
            n273 = call "Concatenate by ref (SubVI).vi"("Response"=w611, "String ref in"=w609) -> ()  [unwired: 9 in, 1 out]
            n274 = call "Concatenate by ref (SubVI).vi"("Response"=w608, "String ref in"=w607) -> ()  [unwired: 9 in, 1 out]
            n275 = call "Concatenate by ref (SubVI).vi"("Response"=w625, "String ref in"=w626) -> ()  [unwired: 9 in, 1 out]
            n276 = Unbundle By Name(w577) -> ("Checksum"=w576:string[])
            n277 = Build Array(w606, w605, w604, w603, w602, w583, w582, w581, w580, w579, w578) -> (w601:bool[])
            n278 = Or Array Elements(Boolean array=w601) -> (logical OR=w546:bool)
            n279 = case shown="True" w546 {
              tunnel: [w631 w634] -> w548
              tunnel: w547 -> [w630 w632]
              frame False {
                n280 = Enqueue Element(queue=w630, element=cluster{"state":string, "element":T1} {"state"="Validate USB", "element"=enum."AUTO"}) -> (error out=w631:errorcluster)  [unwired: 2 in, 2 out]
              }
              frame True {
                n281 = call "Custom two options Message.vi"("MSG"="\n\nNo se pudieron programar todos" ("message"), "Red text"="Abortar", "Green text"="Reintentar") -> ("Ok?"=w633:bool)  [unwired: 8 in]
                n282 = case shown="True" w633 {
                  tunnel: [w638 w642] -> w634
                  tunnel: w632 -> [_ w641]
                  frame False {
                    n283 = xnode "Error Ring"() -> ("error out"=w638:errorcluster)
                  }
                  frame True {
                    n284 = Enqueue Element(queue=w641, element=cluster{"state":string, "element":T1} {"state"="reprogram 2", "element"=enum."AUTO"}) -> (error out=w642:errorcluster)  [unwired: 2 in, 2 out]
                  }
                }
              }
            }
            n285 = Replace Array Subset(array=w576, new element #1=w570, index #1=1 ("index"), new element #2=w569, new element #3=w568, new element #4=w567, new element #5=w566, new element #6=w565, new element #7=w564, new element #8=w563, new element #9=w562, new element #10=w561, new element #11=w560) -> (w574:string[])  [unwired: 10 in]
            n286 = Bundle By Name(cluster=w577, "Checksum"=w574) -> (w575:T3)
          }
          frame "Validate USB" {
            n287 = control-ref of="Status"() -> (w746:refnum<vi>)
            n288 = call "Custom Message.vi"("Boolean Text"="OK", "MSG"="Asegúrese que todos los USB esten conectados" ("message")) -> ()  [unwired: 10 in]
            n289 = call "format console (SubVI).vi"("Caption.Text"="Validación de USB's", "String ref in"=w746) -> ()  [unwired: 9 in, 1 out]
            n290 = Enqueue Element(queue=w736, element=cluster{"state":string, "element":T1} {"state"="PC wait", "element"=enum."AUTO"}) -> (queue out=w740:refnum<queue>, error out=w742:errorcluster)  [unwired: 2 in, 1 out]
            n291 = Enqueue Element(queue=w740, element=cluster{"state":string, "element":T1} {"state"="delay", "element"=enum."AUTO"}, error in (no error)=w742) -> (queue out=w739:refnum<queue>, error out=w741:errorcluster)  [unwired: 1 in, 1 out]
            n292 = Enqueue Element(queue=w739, element=cluster{"state":string, "element":T1} {"state"="Ping", "element"=enum."AUTO"}, error in (no error)=w741) -> (error out=w735:errorcluster)  [unwired: 1 in, 2 out]
            n293 = Bundle By Name(cluster=w733, "USB left"=u16 5) -> (w732:T3)
          }
          frame "PC wait" {
            n294 = control-ref of="Tab Control"() -> (w753:refnum<vi>)
            n295 = control-ref of="Status"() -> (w751:refnum<vi>)
            n296 = property class="TabCtl (strict)"(reference=w753, "Value"=enum32{"Micros", "Micro", "SSH"}."SSH") -> ()  [unwired: 1 in, 2 out]
            n297 = call "format console (SubVI).vi"("Caption.Text"="Esperando a que la computadora inicie", "String ref in"=w751) -> ("String ref out"=w748:refnum<vi>)  [unwired: 9 in]
            n298 = property class="Str"(reference=w748, "Value"="") -> ()  [unwired: 1 in, 2 out]
          }
          frame "delay" {
            n299 = call "Stall Data Flow.vim"("value in"=w755, "milliseconds to wait"=u32 5000) -> ("value out"=w754:T3)  [unwired: 1 out]
          }
          frame "Ping" {
            n300 = control-ref of="Status"() -> (w763:refnum<vi>)
            n301 = call <vilib>:"System Exec.vi"("run minimized? (F)"=TRUE, "working directory"=path "C:/", "command line"="ping -n 4 10.134.246.251") -> ("standard output"=w764:string)  [unwired: 5 in, 3 out]
            n302 = disable-structure "Conditional Disable Structure" shown="RUN_TIME_ENGINE==True&&OS==Win" {
              disable-tunnel: ["perdidos = 0" "Lost = 0"] -> w769
              frame condition #0 (active) {
              }
              frame condition #1 {
              }
            }
            n303 = call "format console (SubVI).vi"("Caption.Text"="Tratando de comunicarse con la PC para empezar el proceso", "String ref in"=w763) -> ("String ref out"=w762:refnum<vi>)  [unwired: 9 in]
            n304 = property on="Tab Control" class="TabCtl (strict)"("Value"=enum32{"Micros", "Micro", "SSH"}."SSH" ("Tab Control")) -> ()  [unwired: 2 in, 2 out]
            n305 = call "Concatenate by ref (SubVI).vi"("Response"=w764, "String ref in"=w762) -> ()  [unwired: 9 in, 1 out]
            n306 = Match Pattern(string=w764, regular expression=w769) -> (offset past match=w770:i32)  [unwired: 1 in, 3 out]
            n307 = Greater Or Equal To 0?(x=w770) -> (x >= 0?=w767:bool)
            n308 = case shown="True" w767 {
              tunnel: w766 -> [w775 w786]
              tunnel: [w778 w781] -> w765
              frame False {
                n309 = Enqueue Element(queue=w775, element=cluster{"state":string, "element":T1} {"state"="delay", "element"=enum."AUTO"}) -> (queue out=w774:refnum<queue>, error out=w773:errorcluster)  [unwired: 2 in, 1 out]
                n310 = Enqueue Element(queue=w774, element=cluster{"state":string, "element":T1} {"state"="Ping", "element"=enum."AUTO"}, error in (no error)=w773) -> (error out=w778:errorcluster)  [unwired: 1 in, 2 out]
              }
              frame True {
                n311 = Enqueue Element(queue=w786, element=cluster{"state":string, "element":T1} {"state"="clear console", "element"=enum."AUTO"}) -> (queue out=w785:refnum<queue>, error out=w783:errorcluster)  [unwired: 2 in, 1 out]
                n312 = disable-structure shown="Enabled" {
                  disable-tunnel: w785 -> [w790 w793]
                  disable-tunnel: w783 -> [w789 w792]
                  disable-tunnel: [w788 w792] -> w782
                  disable-tunnel: [w787 w793] -> w780
                  frame Disabled {
                    n313 = Enqueue Element(queue=w790, element=cluster{"state":string, "element":T1} {"state"="SSH connect", "element"=enum."AUTO"}, error in (no error)=w789) -> (queue out=w787:refnum<queue>, error out=w788:errorcluster)  [unwired: 1 in, 1 out]
                  }
                  frame Enabled {
                  }
                }
                n314 = Enqueue Element(queue=w780, element=cluster{"state":string, "element":T1} {"state"="Clean install", "element"=enum."AUTO"}, error in (no error)=w782) -> (error out=w781:errorcluster)  [unwired: 1 in, 2 out]
              }
            }
            n315 = property on="Parte number" class="Str"() -> ("Value"=w760:string)  [unwired: 2 in, 2 out]
            n316 = Bundle By Name(cluster=w759, "Version"=w760) -> (w758:T3)
          }
          frame "clear console" {
            n317 = control-ref of="Status"() -> (w797:refnum<vi>)
            n318 = property class="Str"(reference=w797, "Value"="") -> ()  [unwired: 1 in, 2 out]
          }
          frame "SSH connect" {
            n319 = Unbundle By Name(w800) -> ("Password"=w799:string)
            n320 = control-ref of="Status"() -> (w806:refnum<vi>)
            n321 = call "format console (SubVI).vi"("Caption.Text"="Conectándose vía TCP-IP con SSH", "String ref in"=w806) -> ()  [unwired: 9 in, 1 out]
            n322 = call "TCP SSH.vi"("States"=T8 "Init", "Password"=w799) -> ("Error  Out"=w804:errorcluster)  [unwired: 7 in, 1 out]
            n323 = case shown="No Error" w804 {
              selector: w804 -> [w811 w813]
              tunnel: w803 -> [_ w819]
              tunnel: w800 -> [w810 w818]
              tunnel: [w809 w817] -> w802
              tunnel: [w811 w812] -> w801
              frame No Error {
                n324 = Bundle By Name(cluster=w810, "Attemps left"=u16 2) -> (w809:T3)
              }
              frame Error {
                n325 = call <vilib>:"Clear Errors.vi"("error in (no error)"=w813) -> ()  [unwired: 5 in, 2 out]
                n326 = Unbundle By Name(w818) -> ("Attemps left"=w815:u16)
                n327 = Less Or Equal To 0?(x=w815) -> (x <= 0?=w814:bool)
                n328 = case shown="True" w814 {
                  tunnel: w819 -> [w822 w823]
                  tunnel: [w820 w828] -> w812
                  frame False {
                    n329 = Enqueue Element(queue=w822, element=cluster{"state":string, "element":T1} {"state"="SSH connect", "element"=enum."AUTO"}) -> (error out=w820:errorcluster)  [unwired: 2 in, 2 out]
                  }
                  frame True {
                    n330 = call "Custom two options Message.vi"("MSG"="El programa no se puede conectar a través de SSH. \nSi desea reintentar asegúrese que la maquina\nEste prendida, y el cable de Ethernet conectado.", "Red text"="Abortar", "Green text"="Reintentar") -> ("Ok?"=w824:bool)  [unwired: 8 in]
                    n331 = case shown="True" w824 {
                      tunnel: [w829 w833] -> w828
                      tunnel: w823 -> [_ w832]
                      frame False {
                        n332 = xnode "Error Ring"() -> ("error out"=w829:errorcluster)
                      }
                      frame True {
                        n333 = Enqueue Element(queue=w832, element=cluster{"state":string, "element":T1} {"state"="SSH connect", "element"=enum."AUTO"}) -> (error out=w833:errorcluster)  [unwired: 2 in, 2 out]
                      }
                    }
                  }
                }
                n334 = Decrement(x=w815) -> (x-1=w816:u16)
                n335 = Bundle By Name(cluster=w818, "Attemps left"=w816) -> (w817:T3)
              }
            }
          }
          frame "Clean install" {
            n336 = Unbundle By Name(w837) -> ("Password"=w835:string)
            n337 = control-ref of="Status"() -> (w839:refnum<vi>)
            n338 = call "SSH Putty.vi"("Command(s) to Execute"="rm -f /*.tar\nrm -rf /usr/jre", "Password"=w835) -> ("error out"=w836:errorcluster)  [unwired: 7 in, 2 out]
            n339 = call "format console (SubVI).vi"("Caption.Text"="Removiendo archivos \".tar\" y la carpeta /usr/jre", "String ref in"=w839) -> ()  [unwired: 9 in, 1 out]
            n340 = Enqueue Element(queue=w842, element=cluster{"state":string, "element":T1} {"state"="File 1 to MI", "element"=enum."AUTO"}, error in (no error)=w836) -> (error out=w841:errorcluster)  [unwired: 1 in, 2 out]
          }
          frame "Clean install Legacy" {
            n341 = call "TCP SSH.vi"("States"=T8 "rm -f /*.tar") -> ("Error  Out"=w852:errorcluster)  [unwired: 8 in, 1 out]
            n342 = control-ref of="Status"() -> (w845:refnum<vi>)
            n343 = call "TCP SSH.vi"("States"=T8 "rm -rf /usr/jre", "Error In"=w852) -> ("Error  Out"=w848:errorcluster)  [unwired: 7 in, 1 out]
            n344 = call "format console (SubVI).vi"("Caption.Text"="Removiendo archivos \".tar\" y la carpeta /usr/jre", "String ref in"=w845) -> ()  [unwired: 9 in, 1 out]
            n345 = Enqueue Element(queue=w849, element=cluster{"state":string, "element":T1} {"state"="File 1 to MI", "element"=enum."AUTO"}, error in (no error)=w848) -> (error out=w847:errorcluster)  [unwired: 1 in, 2 out]
          }
          frame "File 1 to MI" {
            n346 = Unbundle By Name(w866) -> ("Version"=w854:string, "Path: Mi app"=w865:path)
            n347 = Format Into String(format string="%s.tar", w854) -> (resulting string=w857:string)  [unwired: 2 in, 1 out]
            n348 = Format Into String(format string="python send_file_ssh_labview.py /%s.tar %s.tar", w854, w854) -> (resulting string=w853:string)  [unwired: 2 in, 1 out]
            n349 = call <vilib>:"System Exec.vi"("run minimized? (F)"=TRUE, "working directory"=w865, "command line"=w853) -> ("standard output"=w860:string)  [unwired: 5 in, 3 out]
            n350 = Concatenate Strings("Enviando el archivo: " ("Caption.Text"), w857) -> (w856:string)
            n351 = control-ref of="Status"() -> (w862:refnum<vi>)
            n352 = Match Pattern(string=w860, regular expression="File Sent successfully") -> (offset past match=w869:i32)  [unwired: 1 in, 3 out]
            n353 = call "format console (SubVI).vi"("Caption.Text"=w856, "String ref in"=w862) -> ("String ref out"=w861:refnum<vi>)  [unwired: 9 in]
            n354 = Greater Or Equal To 0?(x=w869) -> (x >= 0?=w868:bool)
            n355 = case shown="True" w868 {
              tunnel: [w871 w873] -> w864
              tunnel: w863 -> [_ w875]
              frame False {
                n356 = xnode "Error Ring"() -> ("error out"=w871:errorcluster)
              }
              frame True {
                n357 = Enqueue Element(queue=w875, element=cluster{"state":string, "element":T1} {"state"="File 2 to MI", "element"=enum."AUTO"}) -> (error out=w873:errorcluster)  [unwired: 2 in, 2 out]
              }
            }
            n358 = call "Concatenate by ref (SubVI).vi"("Response"=w860, "String ref in"=w861) -> ()  [unwired: 9 in, 1 out]
          }
          frame "File 2 to MI" {
            n359 = Unbundle By Name(w883) -> ("Path: Mi app"=w882:path)
            n360 = control-ref of="Status"() -> (w878:refnum<vi>)
            n361 = call <vilib>:"System Exec.vi"("run minimized? (F)"=TRUE, "working directory"=w882, "command line"="python send_file_ssh_labview.py /jre.tar.gz jre.tar.gz") -> ("standard output"=w879:string)  [unwired: 5 in, 3 out]
            n362 = call "format console (SubVI).vi"("Caption.Text"="Enviando el archivo: jre.tar.gz", "String ref in"=w878) -> ("String ref out"=w876:refnum<vi>)  [unwired: 9 in]
            n363 = Match Pattern(string=w879, regular expression="File Sent successfully") -> (offset past match=w887:i32)  [unwired: 1 in, 3 out]
            n364 = Greater Or Equal To 0?(x=w887) -> (x >= 0?=w886:bool)
            n365 = call "Concatenate by ref (SubVI).vi"("Response"=w879, "String ref in"=w876) -> ()  [unwired: 9 in, 1 out]
            n366 = case shown="True" w886 {
              tunnel: [w889 w893] -> w881
              tunnel: w880 -> [_ w896]
              frame False {
                n367 = xnode "Error Ring"() -> ("error out"=w889:errorcluster)
              }
              frame True {
                n368 = Enqueue Element(queue=w896, element=cluster{"state":string, "element":T1} {"state"="Check files", "element"=enum."AUTO"}) -> (queue out=w892:refnum<queue>, error out=w894:errorcluster)  [unwired: 2 in, 1 out]
                n369 = Enqueue Element(queue=w892, element=cluster{"state":string, "element":T1} {"state"="clear console", "element"=enum."AUTO"}, error in (no error)=w894) -> (error out=w893:errorcluster)  [unwired: 1 in, 2 out]
              }
            }
          }
          frame "Check files" {
            n370 = Unbundle By Name(w899) -> ("Password"=w898:string)
            n371 = call "SSH Putty.vi"("Command(s) to Execute"="cd /\nls", "Password"=w898) -> ("error out"=w897:errorcluster, "std output"=w900:string)  [unwired: 7 in, 1 out]
            n372 = control-ref of="Status"() -> (w904:refnum<vi>)
            n373 = call "format console (SubVI).vi"("Caption.Text"="Asegurando que los archivos se hayan enviados", "String ref in"=w904) -> ("String ref out"=w902:refnum<vi>)  [unwired: 9 in]
            n374 = call "word finder.vi"("Pattern"="jre.tar.gz", "String"=w900) -> ("finded?"=w909:bool)  [unwired: 9 in]
            n375 = call "word finder.vi"("Pattern"="4.9.12.6034.tar", "String"=w900) -> ("finded?"=w908:bool)  [unwired: 9 in]
            n376 = And(x=w909, y=w908) -> (x .and. y?=w907:bool)
            n377 = call "Concatenate by ref (SubVI).vi"("Response"=w900, "String ref in"=w902) -> ()  [unwired: 9 in, 1 out]
            n378 = case shown="True" w907 {
              tunnel: w906 -> [_ w919]
              tunnel: [w912 w917] -> w905
              tunnel: w897 -> [_ w918]
              frame False {
                n379 = xnode "Error Ring"() -> ("error out"=w912:errorcluster)
              }
              frame True {
                n380 = Enqueue Element(queue=w919, element=cluster{"state":string, "element":T1} {"state"="Send tars", "element"=enum."AUTO"}, error in (no error)=w918) -> (error out=w915:errorcluster)  [unwired: 1 in, 2 out]
                n381 = call "Stall Data Flow.vim"("value in"=w915, "milliseconds to wait"=u32 1000) -> ("value out"=w917:errorcluster)  [unwired: 1 out]
              }
            }
          }
          frame "Check files legacy" {
            n382 = call "TCP SSH.vi"("States"=T8 "cd /") -> ("Error  Out"=w936:errorcluster)  [unwired: 8 in, 1 out]
            n383 = call "TCP SSH.vi"("States"=T8 "ls", "Error In"=w936) -> ("Error  Out"=w934:errorcluster)  [unwired: 7 in, 1 out]
            n384 = call "TCP SSH.vi"("States"=T8 "Read", "Error In"=w934) -> ("Error  Out"=w920:errorcluster, "Response"=w924:string)  [unwired: 7 in]
            n385 = control-ref of="Status"() -> (w923:refnum<vi>)
            n386 = call "format console (SubVI).vi"("Caption.Text"="Asegurando que los archivos se hayan enviados", "String ref in"=w923) -> ("String ref out"=w921:refnum<vi>)  [unwired: 9 in]
            n387 = call "word finder.vi"("Pattern"="jre.tar.gz", "String"=w924) -> ("finded?"=w930:bool)  [unwired: 9 in]
            n388 = call "word finder.vi"("Pattern"="4.9.12.6034.tar", "String"=w924) -> ("finded?"=w929:bool)  [unwired: 9 in]
            n389 = And(x=w930, y=w929) -> (x .and. y?=w928:bool)
            n390 = call "Concatenate by ref (SubVI).vi"("Response"=w924, "String ref in"=w921) -> ()  [unwired: 9 in, 1 out]
            n391 = case shown="True" w928 {
              tunnel: w926 -> [_ w948]
              tunnel: [w938 w945] -> w925
              tunnel: w920 -> [_ w946]
              frame False {
                n392 = xnode "Error Ring"() -> ("error out"=w938:errorcluster)
              }
              frame True {
                n393 = Enqueue Element(queue=w948, element=cluster{"state":string, "element":T1} {"state"="Close SSH", "element"=enum."AUTO"}, error in (no error)=w946) -> (queue out=w943:refnum<queue>, error out=w942:errorcluster)  [unwired: 1 in, 1 out]
                n394 = Enqueue Element(queue=w943, element=cluster{"state":string, "element":T1} {"state"="Send tars", "element"=enum."AUTO"}, error in (no error)=w942) -> (error out=w941:errorcluster)  [unwired: 1 in, 2 out]
                n395 = call "Stall Data Flow.vim"("value in"=w941, "milliseconds to wait"=u32 1000) -> ("value out"=w945:errorcluster)  [unwired: 1 out]
              }
            }
          }
          frame "Send tars" {
            w955 = "\r\n"
            (unwired) "cd /\ntar -xvf 4.9.12.6034.tar\ntar -xvf jre.tar.gz -C /usr" ("Command(s) to Execute")
            n396 = control-ref of="Status"() -> (w964:refnum<vi>)
            n397 = Unbundle By Name(w961) -> ("Version"=w958:string, "Password"=w960:string)
            n398 = Format Into String(format string="tar -xvf %s.tar", w958) -> (resulting string=w956:string)  [unwired: 2 in, 1 out]
            n399 = call "format console (SubVI).vi"("Caption.Text"="Descomprimiendo los archivos enviados", "String ref in"=w964) -> ("String ref out"=w965:refnum<vi>)  [unwired: 9 in]
            n400 = Concatenate Strings("cd /" ("string"), w955, w956, w955, "tar -xvf jre.tar.gz -C /usr") -> (w953:string)
            n401 = call "SSH Putty.vi"("Command(s) to Execute"=w953, "Password"=w960) -> ("error out"=w962:errorcluster, "std output"=w963:string)  [unwired: 7 in, 1 out]
            n402 = call "Concatenate by ref (SubVI).vi"("Response"=w963, "String ref in"=w965) -> ()  [unwired: 9 in, 1 out]
            n403 = Enqueue Element(queue=w951, element=cluster{"state":string, "element":T1} {"state"="clear console", "element"=enum."AUTO"}, error in (no error)=w962) -> (queue out=w950:refnum<queue>, error out=w952:errorcluster)  [unwired: 1 in, 1 out]
            n404 = Enqueue Element(queue=w950, element=cluster{"state":string, "element":T1} {"state"="Search Java", "element"=enum."AUTO"}, error in (no error)=w952) -> (error out=w967:errorcluster)  [unwired: 1 in, 2 out]
          }
          frame "Send tars legacy" {
            n405 = control-ref of="Status"() -> (w981:refnum<vi>)
            n406 = call "TCP SSH.vi"("States"=T8 "tar -xvf 4.9.12.6034.tar") -> ("Error  Out"=w989:errorcluster)  [unwired: 8 in, 1 out]
            n407 = call "format console (SubVI).vi"("Caption.Text"="Descomprimiendo los archivos enviados", "String ref in"=w981) -> ("String ref out"=w982:refnum<vi>)  [unwired: 9 in]
            n408 = call "TCP SSH.vi"("States"=T8 "Read", "Error In"=w989) -> ("Error  Out"=w988:errorcluster, "Response"=w986:string)  [unwired: 7 in]
            n409 = call "Concatenate by ref (SubVI).vi"("Response"=w986, "String ref in"=w982) -> ("String ref off"=w984:refnum<vi>)  [unwired: 9 in]
            n410 = call "Stall Data Flow.vim"("value in"=w988, "milliseconds to wait"=u32 15000) -> ("value out"=w970:errorcluster)  [unwired: 1 out]
            n411 = call "TCP SSH.vi"("States"=T8 "tar -xvf jre.tar.gz -C /usr", "Error In"=w970) -> ("Error  Out"=w987:errorcluster)  [unwired: 7 in, 1 out]
            n412 = call "TCP SSH.vi"("States"=T8 "Read", "Error In"=w987) -> ("Error  Out"=w977:errorcluster, "Response"=w985:string)  [unwired: 7 in]
            n413 = call "Concatenate by ref (SubVI).vi"("Response"=w985, "String ref in"=w984) -> ()  [unwired: 9 in, 1 out]
            n414 = Enqueue Element(queue=w976, element=cluster{"state":string, "element":T1} {"state"="Close SSH", "element"=enum."AUTO"}, error in (no error)=w977) -> (queue out=w971:refnum<queue>, error out=w972:errorcluster)  [unwired: 1 in, 1 out]
            n415 = Enqueue Element(queue=w971, element=cluster{"state":string, "element":T1} {"state"="SSH connect", "element"=enum."AUTO"}, error in (no error)=w972) -> (queue out=w975:refnum<queue>, error out=w978:errorcluster)  [unwired: 1 in, 1 out]
            n416 = Enqueue Element(queue=w975, element=cluster{"state":string, "element":T1} {"state"="Search Java", "element"=enum."AUTO"}, error in (no error)=w978) -> (error out=w990:errorcluster)  [unwired: 1 in, 2 out]
          }
          frame "Search Java" {
            w995 = "1.8.0-b132" ("regular expression")
            n417 = Unbundle By Name(w997) -> ("Password"=w998:string)
            n418 = control-ref of="Status"() -> (w1001:refnum<vi>)
            n419 = call "SSH Putty.vi"("Command(s) to Execute"="/usr/jre/bin/java -version", "Password"=w998) -> ("std error"=w1005:string, "std output"=w1004:string)  [unwired: 7 in, 1 out]
            n420 = Concatenate Strings(w1004, w1005) -> (w999:string)
            n421 = call "format console (SubVI).vi"("Caption.Text"="Asegurando que la version de java sea la correcta", "String ref in"=w1001) -> ("String ref out"=w1002:refnum<vi>)  [unwired: 9 in]
            n422 = call "word finder.vi"("Pattern"=w995, "String"=w999) -> ("finded?"=w1003:bool)  [unwired: 9 in]
            n423 = call "Concatenate by ref (SubVI).vi"("Response"=w999, "String ref in"=w1002) -> ()  [unwired: 9 in, 1 out]
            n424 = case shown="True" w1003 {
              tunnel: [w1009 w1022] -> w1008
              tunnel: w1007 -> [_ w1016]
              frame False {
                n425 = xnode "Error Ring"() -> ("error out"=w1009:errorcluster)
              }
              frame True {
                n426 = Enqueue Element(queue=w1016, element=cluster{"state":string, "element":T1} {"state"="clear console", "element"=enum."AUTO"}) -> (queue out=w1020:refnum<queue>, error out=w1019:errorcluster)  [unwired: 2 in, 1 out]
                n427 = disable-structure shown="Enabled" {
                  disable-tunnel: w1020 -> [w1027 w1029]
                  disable-tunnel: w1019 -> [w1026 w1028]
                  disable-tunnel: [w1025 w1028] -> w1017
                  disable-tunnel: [w1024 w1029] -> w1015
                  frame Disabled {
                    n428 = Enqueue Element(queue=w1027, element=cluster{"state":string, "element":T1} {"state"="SSH connect", "element"=enum."AUTO"}, error in (no error)=w1026) -> (queue out=w1024:refnum<queue>, error out=w1025:errorcluster)  [unwired: 1 in, 1 out]
                  }
                  frame Enabled {
                  }
                }
                n429 = Enqueue Element(queue=w1015, element=cluster{"state":string, "element":T1} {"state"="Kill all", "element"=enum."AUTO"}, error in (no error)=w1017) -> (error out=w1022:errorcluster)  [unwired: 1 in, 2 out]
              }
            }
            n430 = Bundle By Name(cluster=w997, "Java"=w995) -> (w996:T3)
          }
          frame "Kill all" {
            n431 = Unbundle By Name(w1032) -> ("Password"=w1031:string)
            n432 = call "SSH Putty.vi"("Command(s) to Execute"="cd /\nrm -f /*.tar\nrm -f /*.gz\nkillall MonitorDaemon.exe\nkillall java\nkillall WIFIAgent.exe\nkillall DataProcessor.exe\ncp -rf rootfs/* /", "Password"=w1031) -> ("error out"=w1030:errorcluster)  [unwired: 7 in, 2 out]
            n433 = control-ref of="Status"() -> (w1037:refnum<vi>)
            n434 = call "format console (SubVI).vi"("Caption.Text"="Terminando procesos (.exe)", "String ref in"=w1037) -> ()  [unwired: 9 in, 1 out]
            n435 = call "Stall Data Flow.vim"("value in"=w1030, "milliseconds to wait"=u32 1000) -> ("value out"=w1035:errorcluster)  [unwired: 1 out]
            n436 = Enqueue Element(queue=w1040, element=cluster{"state":string, "element":T1} {"state"="Sync", "element"=enum."AUTO"}, error in (no error)=w1035) -> (error out=w1038:errorcluster)  [unwired: 1 in, 2 out]
          }
          frame "Kill all legacy" {
            n437 = call "TCP SSH.vi"("States"=T8 "cd /") -> ("Error  Out"=w1044:errorcluster)  [unwired: 8 in, 1 out]
            n438 = call "TCP SSH.vi"("States"=T8 "rm -f /*.tar", "Error In"=w1044) -> ("Error  Out"=w1054:errorcluster)  [unwired: 7 in, 1 out]
            n439 = call "TCP SSH.vi"("States"=T8 "rm -f /*.gz", "Error In"=w1054) -> ("Error  Out"=w1056:errorcluster)  [unwired: 7 in, 1 out]
            n440 = control-ref of="Status"() -> (w1046:refnum<vi>)
            n441 = call "TCP SSH.vi"("States"=T8 "killall DataProcessor.exe", "Error In"=w1056) -> ("Error  Out"=w1057:errorcluster)  [unwired: 7 in, 1 out]
            n442 = call "format console (SubVI).vi"("Caption.Text"="Terminando procesos (.exe)", "String ref in"=w1046) -> ()  [unwired: 9 in, 1 out]
            n443 = call "TCP SSH.vi"("States"=T8 "killall WIFIAgent.exe", "Error In"=w1057) -> ("Error  Out"=w1059:errorcluster)  [unwired: 7 in, 1 out]
            n444 = call "TCP SSH.vi"("States"=T8 "killall java", "Error In"=w1059) -> ("Error  Out"=w1061:errorcluster)  [unwired: 7 in, 1 out]
            n445 = call "TCP SSH.vi"("States"=T8 "killall MonitorDaemon.exe", "Error In"=w1061) -> ("Error  Out"=w1047:errorcluster)  [unwired: 7 in, 1 out]
            n446 = call "Stall Data Flow.vim"("value in"=w1047, "milliseconds to wait"=u32 1000) -> ("value out"=w1042:errorcluster)  [unwired: 1 out]
            n447 = Enqueue Element(queue=w1050, element=cluster{"state":string, "element":T1} {"state"="Copy rootfs", "element"=enum."AUTO"}, error in (no error)=w1042) -> (error out=w1048:errorcluster)  [unwired: 1 in, 2 out]
          }
          frame "Copy rootfs" {
            n448 = control-ref of="Status"() -> (w1066:refnum<vi>)
            n449 = call "format console (SubVI).vi"("Caption.Text"="Copiando archivos de rootfs/*, a:  /", "String ref in"=w1066) -> ()  [unwired: 9 in, 1 out]
            n450 = call "TCP SSH.vi"("States"=T8 "cp -rf rootfs/* /") -> ("Error  Out"=w1070:errorcluster)  [unwired: 8 in, 1 out]
            n451 = call "Stall Data Flow.vim"("value in"=w1070, "milliseconds to wait"=u32 1000) -> ("value out"=w1064:errorcluster)  [unwired: 1 out]
            n452 = Enqueue Element(queue=w1068, element=cluster{"state":string, "element":T1} {"state"="Sync", "element"=enum."AUTO"}, error in (no error)=w1064) -> (error out=w1069:errorcluster)  [unwired: 1 in, 2 out]
          }
          frame "Sync" {
            n453 = Unbundle By Name(w1076) -> ("Password"=w1074:string)
            n454 = call "SSH Putty.vi"("Command(s) to Execute"="sync", "Password"=w1074) -> ("error out"=w1075:errorcluster)  [unwired: 7 in, 2 out]
            n455 = control-ref of="Status"() -> (w1083:refnum<vi>)
            n456 = call "Stall Data Flow.vim"("value in"=w1075, "milliseconds to wait"=u32 3000) -> ("value out"=w1078:errorcluster)  [unwired: 1 out]
            n457 = call "format console (SubVI).vi"("Caption.Text"="Sincronizando", "String ref in"=w1083) -> ()  [unwired: 9 in, 1 out]
            n458 = Enqueue Element(queue=w1086, element=cluster{"state":string, "element":T1} {"state"="clear console", "element"=enum."AUTO"}, error in (no error)=w1078) -> (queue out=w1080:refnum<queue>, error out=w1079:errorcluster)  [unwired: 1 in, 1 out]
            n459 = Enqueue Element(queue=w1080, element=cluster{"state":string, "element":T1} {"state"="SED", "element"=enum."AUTO"}, error in (no error)=w1079) -> (error out=w1085:errorcluster)  [unwired: 1 in, 2 out]
          }
          frame "Sync legacy" {
            n460 = control-ref of="Status"() -> (w1094:refnum<vi>)
            n461 = call "format console (SubVI).vi"("Caption.Text"="Sincronizando", "String ref in"=w1094) -> ()  [unwired: 9 in, 1 out]
            n462 = call "TCP SSH.vi"("States"=T8 "sync") -> ("Error  Out"=w1091:errorcluster)  [unwired: 8 in, 1 out]
            n463 = call "Stall Data Flow.vim"("value in"=w1091, "milliseconds to wait"=u32 1000) -> ("value out"=w1088:errorcluster)  [unwired: 1 out]
            n464 = Enqueue Element(queue=w1097, element=cluster{"state":string, "element":T1} {"state"="clear console", "element"=enum."AUTO"}, error in (no error)=w1088) -> (queue out=w1090:refnum<queue>, error out=w1089:errorcluster)  [unwired: 1 in, 1 out]
            n465 = Enqueue Element(queue=w1090, element=cluster{"state":string, "element":T1} {"state"="SED", "element"=enum."AUTO"}, error in (no error)=w1089) -> (error out=w1096:errorcluster)  [unwired: 1 in, 2 out]
          }
          frame "Flush" {
            n466 = while {
              tunnel: [w1104] -> w1100
              stop <- w1105 stop-if-true
              n467 = control-ref of="Status"() -> (w1103:refnum<vi>)
              n468 = call "TCP SSH.vi"("States"=T8 "Read") -> ("Error  Out"=w1104:errorcluster, "Response"=w1102:string)  [unwired: 8 in]
              n469 = Empty String/Path?(string/path=w1102) -> (empty?=w1105:bool)
              n470 = call "Concatenate by ref (SubVI).vi"("Response"=w1102, "String ref in"=w1103) -> ()  [unwired: 9 in, 1 out]
            }
          }
          frame "SED" {
            w1111 = "https://13.248.167.220/metadata"
            n471 = Unbundle By Name(w1109) -> ("Password"=w1108:string)
            n472 = control-ref of="Status"() -> (w1115:refnum<vi>)
            n473 = call "SSH Putty.vi"("Command(s) to Execute"="cd /\ncd hdplus\nsed -i 's/^REMOTE_CONFIG_URL_TEMPLATE=.*/REMOTE_CONFIG_URL_TEMPLATE=https:\\/\\/13.248.167.220\\/metadata\\/%s/g' /hdplus/tablo.conf\ncat /hdplus/tablo.conf", "Password"=w1108) -> ("std output"=w1107:string)  [unwired: 7 in, 2 out]
            n474 = call "format console (SubVI).vi"("Caption.Text"="Buscando la palabra \"https://13.248.167.220/metadata\"", "String ref in"=w1115) -> ("String ref out"=w1113:refnum<vi>)  [unwired: 9 in]
            n475 = call "word finder.vi"("Pattern"=w1111, "String"=w1107) -> ("finded?"=w1116:bool)  [unwired: 9 in]
            n476 = call "Concatenate by ref (SubVI).vi"("String ref in"=w1113) -> ()  [unwired: 10 in, 1 out]
            n477 = case shown="True" w1116 {
              tunnel: [w1119 w1122] -> w1118
              tunnel: w1117 -> [_ w1124]
              frame False {
                n478 = xnode "Error Ring"() -> ("error out"=w1119:errorcluster)
              }
              frame True {
                n479 = Enqueue Element(queue=w1124, element=cluster{"state":string, "element":T1} {"state"="Telnet", "element"=enum."AUTO"}) -> (error out=w1125:errorcluster)  [unwired: 2 in, 2 out]
                n480 = call "Stall Data Flow.vim"("value in"=w1125, "milliseconds to wait"=u32 3000) -> ("value out"=w1122:errorcluster)  [unwired: 1 out]
              }
            }
            n481 = Bundle By Name(cluster=w1109, "URL"=w1111) -> (w1112:T3)
          }
          frame "SED Legacy" {
            w1126 = "https://13.248.167.220/metadata"
            n482 = call "TCP SSH.vi"("States"=T8 "cd hdplus") -> ("Error  Out"=w1142:errorcluster)  [unwired: 8 in, 1 out]
            n483 = call "TCP SSH.vi"("States"=T8 "sed -i", "Error In"=w1142) -> ("Error  Out"=w1144:errorcluster)  [unwired: 7 in, 1 out]
            n484 = control-ref of="Status"() -> (w1134:refnum<vi>)
            n485 = call "TCP SSH.vi"("States"=T8 "cat /hdplus/tablo.conf", "Error In"=w1144) -> ("Error  Out"=w1137:errorcluster)  [unwired: 7 in, 1 out]
            n486 = call "format console (SubVI).vi"("Caption.Text"="Buscando la palabra \"https://13.248.167.220/metadata\"", "String ref in"=w1134) -> ("String ref out"=w1132:refnum<vi>)  [unwired: 9 in]
            n487 = call "Stall Data Flow.vim"("value in"=w1137, "milliseconds to wait"=u32 15000) -> ("value out"=w1130:errorcluster)  [unwired: 1 out]
            n488 = call "TCP SSH.vi"("States"=T8 "Read", "Error In"=w1130) -> ("Response"=w1131:string)  [unwired: 7 in, 1 out]
            n489 = call "word finder.vi"("Pattern"=w1126, "String"=w1131) -> ("finded?"=w1135:bool)  [unwired: 9 in]
            n490 = call "Concatenate by ref (SubVI).vi"("Response"=w1131, "String ref in"=w1132) -> ()  [unwired: 9 in, 1 out]
            n491 = case shown="True" w1135 {
              tunnel: [w1145 w1149] -> w1139
              tunnel: w1138 -> [_ w1148]
              frame False {
                n492 = xnode "Error Ring"() -> ("error out"=w1145:errorcluster)
              }
              frame True {
                n493 = Enqueue Element(queue=w1148, element=cluster{"state":string, "element":T1} {"state"="Telnet", "element"=enum."AUTO"}) -> (error out=w1149:errorcluster)  [unwired: 2 in, 2 out]
              }
            }
            n494 = Bundle By Name(cluster=w1128, "URL"=w1126) -> (w1127:T3)
          }
          frame "Telnet" {
            n495 = Unbundle By Name(w1153) -> ("Password"=w1152:string)
            n496 = control-ref of="Status"() -> (w1157:refnum<vi>)
            n497 = call "SSH Putty.vi"("Command(s) to Execute"="cd /\ncd hdplus\nscript/disableTelnet", "Password"=w1152) -> ("error out"=w1150:errorcluster, "std output"=w1151:string)  [unwired: 7 in, 1 out]
            n498 = call "format console (SubVI).vi"("Caption.Text"="Deshabilitando Telnet", "String ref in"=w1157) -> ("String ref out"=w1155:refnum<vi>)  [unwired: 9 in]
            n499 = call "Concatenate by ref (SubVI).vi"("Response"=w1151, "String ref in"=w1155) -> ()  [unwired: 9 in, 1 out]
            n500 = call "word finder.vi"("Pattern"="Telnet confirmed disabled", "String"=w1151) -> ("finded?"=w1159:bool)  [unwired: 9 in]
            n501 = case shown="True" w1159 {
              tunnel: [w1162 w1167] -> w1161
              tunnel: w1150 -> [_ w1164]
              tunnel: w1158 -> [_ w1165]
              frame False {
                n502 = xnode "Error Ring"() -> ("error out"=w1162:errorcluster)
              }
              frame True {
                n503 = Enqueue Element(queue=w1165, element=cluster{"state":string, "element":T1} {"state"="Search Data", "element"=enum."AUTO"}, error in (no error)=w1164) -> (error out=w1167:errorcluster)  [unwired: 1 in, 2 out]
              }
            }
          }
          frame "Telnet legacy" {
            n504 = control-ref of="Status"() -> (w1171:refnum<vi>)
            n505 = call "TCP SSH.vi"("States"=T8 "script/disableTelnet") -> ("Error  Out"=w1176:errorcluster)  [unwired: 8 in, 1 out]
            n506 = call "format console (SubVI).vi"("Caption.Text"="Deshabilitando Telnet", "String ref in"=w1171) -> ("String ref out"=w1169:refnum<vi>)  [unwired: 9 in]
            n507 = call "TCP SSH.vi"("States"=T8 "Read", "Error In"=w1176) -> ("Error  Out"=w1175:errorcluster, "Response"=w1168:string)  [unwired: 7 in]
            n508 = call "Concatenate by ref (SubVI).vi"("Response"=w1168, "String ref in"=w1169) -> ()  [unwired: 9 in, 1 out]
            n509 = call "word finder.vi"("Pattern"="Telnet confirmed disabled", "String"=w1168) -> ("finded?"=w1173:bool)  [unwired: 9 in]
            n510 = case shown="True" w1173 {
              tunnel: [w1181 w1186] -> w1178
              tunnel: w1175 -> [_ w1184]
              tunnel: w1172 -> [_ w1183]
              frame False {
                n511 = xnode "Error Ring"() -> ("error out"=w1181:errorcluster)
              }
              frame True {
                n512 = Enqueue Element(queue=w1183, element=cluster{"state":string, "element":T1} {"state"="Search Data", "element"=enum."AUTO"}, error in (no error)=w1184) -> (error out=w1186:errorcluster)  [unwired: 1 in, 2 out]
              }
            }
          }
          frame "Search Data" {
            n513 = Unbundle By Name(w1189) -> ("Password"=w1188:string)
            n514 = control-ref of="Status"() -> (w1200:refnum<vi>)
            n515 = call "SSH Putty.vi"("Command(s) to Execute"="cd /\ncd hdplus\nls", "Password"=w1188) -> ("error out"=w1190:errorcluster, "std output"=w1187:string)  [unwired: 7 in, 1 out]
            n516 = call "format console (SubVI).vi"("Caption.Text"="Buscando el archivo: DataProcessor.exe", "String ref in"=w1200) -> ("String ref out"=w1198:refnum<vi>)  [unwired: 9 in]
            n517 = call "Concatenate by ref (SubVI).vi"("Response"=w1187, "String ref in"=w1198) -> ()  [unwired: 9 in, 1 out]
            n518 = Match Pattern(string=w1187, regular expression="DataProcessor.exe") -> (offset past match=w1203:i32)  [unwired: 1 in, 3 out]
            n519 = Greater Or Equal To 0?(x=w1203) -> (x >= 0?=w1195:bool)
            n520 = case shown="True" w1195 {
              tunnel: [w1204 w1215] -> w1202
              tunnel: w1201 -> [_ w1208]
              tunnel: w1190 -> [_ w1213]
              frame False {
                n521 = xnode "Error Ring"() -> ("error out"=w1204:errorcluster)
              }
              frame True {
                n522 = Enqueue Element(queue=w1208, element=cluster{"state":string, "element":T1} {"state"="SSH connect", "element"=enum."AUTO"}, error in (no error)=w1213) -> (queue out=w1209:refnum<queue>, error out=w1212:errorcluster)  [unwired: 1 in, 1 out]
                n523 = Enqueue Element(queue=w1209, element=cluster{"state":string, "element":T1} {"state"="delay", "element"=enum."AUTO"}, error in (no error)=w1212) -> (queue out=w1210:refnum<queue>, error out=w1211:errorcluster)  [unwired: 1 in, 1 out]
                n524 = Enqueue Element(queue=w1210, element=cluster{"state":string, "element":T1} {"state"="Dev", "element"=enum."AUTO"}, error in (no error)=w1211) -> (error out=w1215:errorcluster)  [unwired: 1 in, 2 out]
              }
            }
            n525 = Select(t="True", s=w1195, f="False") -> (s? t:f=w1192:string)
            n526 = Bundle By Name(cluster=w1189, "DataProcessor?"=w1192) -> (w1196:T3)
          }
          frame "Search Data legacy" {
            n527 = call "TCP SSH.vi"("States"=T8 "ls") -> ("Error  Out"=w1230:errorcluster)  [unwired: 8 in, 1 out]
            n528 = control-ref of="Status"() -> (w1226:refnum<vi>)
            n529 = call "TCP SSH.vi"("States"=T8 "Read", "Error In"=w1230) -> ("Response"=w1222:string)  [unwired: 7 in, 1 out]
            n530 = call "format console (SubVI).vi"("Caption.Text"="Buscando el archivo: DataProcessor.exe", "String ref in"=w1226) -> ("String ref out"=w1224:refnum<vi>)  [unwired: 9 in]
            n531 = call "Concatenate by ref (SubVI).vi"("Response"=w1222, "String ref in"=w1224) -> ()  [unwired: 9 in, 1 out]
            n532 = Match Pattern(string=w1222, regular expression="DataProcessor.exe") -> (offset past match=w1232:i32)  [unwired: 1 in, 3 out]
            n533 = Greater Or Equal To 0?(x=w1232) -> (x >= 0?=w1219:bool)
            n534 = case shown="True" w1219 {
              tunnel: [w1233 w1237] -> w1229
              tunnel: w1228 -> [_ w1236]
              frame False {
                n535 = xnode "Error Ring"() -> ("error out"=w1233:errorcluster)
              }
              frame True {
                n536 = Enqueue Element(queue=w1236, element=cluster{"state":string, "element":T1} {"state"="Dev", "element"=enum."AUTO"}) -> (error out=w1237:errorcluster)  [unwired: 2 in, 2 out]
              }
            }
            n537 = Select(t="True", s=w1219, f="False") -> (s? t:f=w1216:string)
            n538 = Bundle By Name(cluster=w1221, "DataProcessor?"=w1216) -> (w1220:T3)
          }
          frame "Dev" {
            n539 = call "TCP SSH.vi"("States"=T8 "cd /dev") -> ("Error  Out"=w1241:errorcluster)  [unwired: 8 in, 1 out]
            n540 = Enqueue Element(queue=w1239, element=cluster{"state":string, "element":T1} {"state"="Check USB", "element"=enum."AUTO"}, error in (no error)=w1241) -> (error out=w1240:errorcluster)  [unwired: 1 in, 2 out]
          }
          frame "Check USB" {
            w1244 = u16 5 ("x")
            n541 = call "TCP SSH.vi"("States"=T8 "ls sd*") -> ("Error  Out"=w1250:errorcluster)  [unwired: 8 in, 1 out]
            n542 = call "TCP SSH.vi"("States"=T8 "Read", "Error In"=w1250) -> ("Response"=w1248:string)  [unwired: 7 in, 1 out]
            n543 = control-ref of="Status"() -> (w1253:refnum<vi>)
            n544 = call "string pattern counter.vi"("pattern"="sd", "string"=w1248) -> ("Numeric"=w1247:u16)  [unwired: 9 in]
            n545 = Equal?(x=w1244, y=w1247) -> (x = y?=w1245:bool)
            n546 = case shown="False" w1245 {
              tunnel: w1256 -> [w1267 w1273]
              tunnel: [w1266 w1274] -> w1254
              tunnel: w1247 -> [w1265 _]
              tunnel: w1244 -> [w1257 _]
              frame False {
                n547 = Format Into String(format string="Se contaron %d USB montada(s), \ny deberian ser %d", w1265, w1257) -> (resulting string=w1259:string)  [unwired: 2 in, 1 out]
                n548 = Concatenate Strings("\n" ("string"), w1259) -> (w1258:string)
                n549 = call "Custom two options Message.vi"("MSG"=w1258, "Red text"="Abortar" ("F button name (\"Cancel\")"), "Green text"="Reintentar" ("T button name (\"OK\")")) -> ("Ok?"=w1261:bool)  [unwired: 8 in]
                n550 = case shown="True" w1261 {
                  tunnel: w1267 -> [_ w1272]
                  tunnel: [w1268 w1270] -> w1266
                  frame False {
                    n551 = xnode "Error Ring"() -> ("error out"=w1268:errorcluster)
                  }
                  frame True {
                    n552 = Enqueue Element(queue=w1272, element=cluster{"state":string, "element":T1} {"state"="Check USB", "element"=enum."AUTO"}) -> (error out=w1270:errorcluster)  [unwired: 2 in, 2 out]
                  }
                }
              }
              frame True {
                n553 = Enqueue Element(queue=w1273, element=cluster{"state":string, "element":T1} {"state"="Close SSH", "element"=enum."AUTO"}) -> (queue out=w1276:refnum<queue>, error out=w1277:errorcluster)  [unwired: 2 in, 1 out]
                n554 = Enqueue Element(queue=w1276, element=cluster{"state":string, "element":T1} {"state"="End", "element"=enum."AUTO"}, error in (no error)=w1277) -> (error out=w1274:errorcluster)  [unwired: 1 in, 2 out]
              }
            }
            n555 = call "format console (SubVI).vi"("Caption.Text"="Validación con USB's", "String ref in"=w1253) -> ()  [unwired: 9 in, 1 out]
          }
          frame "Check 5 USB - Legacy" {
            n556 = Unbundle By Name(w1285) -> ("USB left"=w1283:u16)
            n557 = Increment(x=w1283) -> (x+1=w1279:u16)
            n558 = Less Or Equal To 0?(x=w1279) -> (x <= 0?=w1287:bool)
            n559 = case shown="False" w1287 {
              tunnel: w1283 -> [w1288 _]
              tunnel: w1286 -> [w1298 w1345]
              tunnel: w1285 -> [w1296 w1343]
              tunnel: [w1295 w1343] -> w1284
              tunnel: w1283 -> [w1294 _]
              tunnel: [w1293 w1341] -> w1282
              frame False {
                n560 = call "TCP SSH.vi"("States"=T8 "ls sd*") -> ("Error  Out"=w1301:errorcluster)  [unwired: 8 in, 1 out]
                n561 = Greater?(x=w1288, y=u16 1) -> (0:w1291:bool)
                n562 = case shown="True" w1291 {
                  tunnel: ["Quite la ultima USB" ("format string") w1305] -> w1290
                  tunnel: w1288 -> [_ w1306]
                  frame False {
                  }
                  frame True {
                    n563 = Format Into String(format string="Quite una de las %d USB montadas", w1306) -> (resulting string=w1305:string)  [unwired: 2 in, 1 out]
                  }
                }
                n564 = call "TCP SSH.vi"("States"=T8 "Read", "Error In"=w1301) -> ("Response"=w1299:string)  [unwired: 7 in, 1 out]
                n565 = call "string pattern counter.vi"("pattern"="sd", "string"=w1299) -> ("Numeric"=w1297:u16)  [unwired: 9 in]
                n566 = Equal?(x=w1288, y=w1297) -> (x = y?=w1302:bool)
                n567 = case shown="True" w1302 {
                  tunnel: w1290 -> [_ w1327]
                  tunnel: w1298 -> [w1316 w1334]
                  tunnel: w1297 -> [w1318 _]
                  tunnel: w1296 -> [w1317 w1332]
                  tunnel: [w1317 w1331] -> w1295
                  tunnel: w1294 -> [_ w1330]
                  tunnel: [w1315 w1328] -> w1293
                  tunnel: w1288 -> [w1311 _]
                  tunnel: w1288 -> [_ w1325]
                  frame False {
                    n568 = Format Into String(format string="Se contaron %d USB montada(s), \ny deberian ser %d", w1318, w1311) -> (resulting string=w1309:string)  [unwired: 2 in, 1 out]
                    n569 = Concatenate Strings("\n" ("string"), w1309) -> (w1308:string)
                    n570 = call "Custom two options Message.vi"("MSG"=w1308, "Red text"="Abortar" ("F button name (\"Cancel\")"), "Green text"="Reintentar" ("T button name (\"OK\")")) -> ("Ok?"=w1312:bool)  [unwired: 8 in]
                    n571 = case shown="False" w1312 {
                      tunnel: w1316 -> [_ w1324]
                      tunnel: [w1320 w1322] -> w1315
                      frame False {
                        n572 = xnode "Error Ring"() -> ("error out"=w1320:errorcluster)
                      }
                      frame True {
                        n573 = Enqueue Element(queue=w1324, element=cluster{"state":string, "element":T1} {"state"="Check USB", "element"=enum."AUTO"}) -> (error out=w1322:errorcluster)  [unwired: 2 in, 2 out]
                      }
                    }
                  }
                  frame True {
                    n574 = Greater Than 0?(x=w1325) -> (x > 0?=w1326:bool)
                    n575 = case shown="True" w1326 {
                      tunnel: w1327 -> [_ w1337]
                      frame False {
                      }
                      frame True {
                        n576 = Concatenate Strings("\n\n" ("string"), w1337) -> (w1335:string)
                        n577 = call "Custom Message.vi"("Boolean Text"="OK", "MSG"=w1335) -> ()  [unwired: 10 in]
                      }
                    }
                    n578 = Decrement(x=w1330) -> (x-1=w1329:u16)
                    n579 = Enqueue Element(queue=w1334, element=cluster{"state":string, "element":T1} {"state"="Check USB", "element"=enum."AUTO"}) -> (error out=w1328:errorcluster)  [unwired: 2 in, 2 out]
                    n580 = Bundle By Name(cluster=w1332, "USB left"=w1329) -> (w1331:T3)
                  }
                }
              }
              frame True {
                n581 = Enqueue Element(queue=w1345, element=cluster{"state":string, "element":T1} {"state"="Close SSH", "element"=enum."AUTO"}) -> (queue out=w1340:refnum<queue>, error out=w1342:errorcluster)  [unwired: 2 in, 1 out]
                n582 = Enqueue Element(queue=w1340, element=cluster{"state":string, "element":T1} {"state"="End", "element"=enum."AUTO"}, error in (no error)=w1342) -> (error out=w1341:errorcluster)  [unwired: 1 in, 2 out]
              }
            }
            n583 = control-ref of="Status"() -> (w1281:refnum<vi>)
            n584 = call "format console (SubVI).vi"("Caption.Text"="Validación con USB's", "String ref in"=w1281) -> ()  [unwired: 9 in, 1 out]
          }
          frame "Close SSH" {
            n585 = call "TCP SSH.vi"("States"=T8 "Close") -> ("Error  Out"=w1347:errorcluster)  [unwired: 8 in, 1 out]
          }
          frame "End" {
            n586 = Unbundle By Name(w1355) -> ("Checksum"=w1349:string[], "ID"=w1354:string, "Version"=w1353:string, "Java"=w1352:string, "URL"=w1351:string, "DataProcessor?"=w1350:string)
            n587 = control-ref of="Tab Control"() -> (w1362:refnum<vi>)
            n588 = call "Custom Message.vi"("MSG"="\n¡Proceso terminado con exito!") -> ()  [unwired: 11 in]
            n589 = property class="TabCtl (strict)"(reference=w1362, "Value"=enum32{"Micros", "Micro", "SSH"}."Micro") -> ()  [unwired: 1 in, 2 out]
            n590 = call "Log File.vi"("Version"=w1353, "ID"=w1354, "Checksums"=w1349, "Java"=w1352, "URL"=w1351, "DataProcessor.exe?"=w1350, "Pass?"="True", "Error"="") -> ()  [unwired: 7 in, 1 out]
            n591 = property on="Pass or fail" class="Str"("Value"="TEST PASSED" ("Pass or fail"), "Text.BGColor"=u32 6618880 ("Text.Text Colors:BG Color"), "Text.FontSize"=u32 163 ("Text.Font:Size")) -> ()  [unwired: 2 in, 2 out]
            n592 = property on="Start Button" class="Bool (strict)"("Val(Sgnl)"=FALSE ("Start Button")) -> (error out=w1364:errorcluster)  [unwired: 2 in, 1 out]
          }
        }
      }
      frame Error {
        n593 = Unbundle By Name(w1380) -> ("source"=w1367:string)
        n594 = Unbundle By Name(w1368) -> ("Checksum"=w1366:string[], "ID"=w1373:string, "Version"=w1372:string, "Java"=w1371:string, "URL"=w1370:string, "DataProcessor?"=w1369:string)
        n595 = call <vilib>:"Clear Errors.vi"("error in (no error)"=w1380) -> ("error out"=w1383:errorcluster)  [unwired: 5 in, 1 out]
        n596 = Concatenate Strings("\r\n", w1367) -> (w1381:string)
        n597 = call "TCP SSH.vi"("States"=T8 "Close", "Error In"=w1383) -> ("Error  Out"=w1384:errorcluster)  [unwired: 7 in, 1 out]
        n598 = call "Custom Error Message.vi"("MSG"=w1381) -> ()  [unwired: 11 in]
        n599 = Flush Queue(queue=w1392, error in (no error)=w1383) -> (queue out=w1390:refnum<queue>, error out=w1391:errorcluster)  [unwired: 1 out]
        n600 = call "Log File.vi"("Version"=w1372, "ID"=w1373, "Checksums"=w1366, "Java"=w1371, "URL"=w1370, "DataProcessor.exe?"=w1369, "Pass?"="False", "Error"=w1367) -> ()  [unwired: 7 in, 1 out]
        n601 = call <vilib>:"Clear Errors.vi"("error in (no error)"=w1384) -> ()  [unwired: 5 in, 2 out]
        n602 = Enqueue Element(queue=w1390, element=cluster{"state":string, "element":T1} {"state"="idle", "element"=enum."AUTO"}, error in (no error)=w1391) -> (error out=w1387:errorcluster)  [unwired: 1 in, 2 out]
        n603 = control-ref of="Tab Control"() -> (w1376:refnum<vi>)
        n604 = property class="TabCtl (strict)"(reference=w1376, "Value"=enum32{"Micros", "Micro", "SSH"}."Micro") -> ()  [unwired: 1 in, 2 out]
        n605 = property on="Pass or fail" class="Str"("Value"="TEST FAILED" ("Pass or fail"), "Text.BGColor"=u32 16711680 ("Text.Text Colors:BG Color"), "Text.FontSize"=u32 163 ("Text.Font:Size")) -> ()  [unwired: 2 in, 2 out]
        n606 = property on="Start Button" class="Bool (strict)"(error in=w1387, "Val(Sgnl)"=FALSE ("Start Button")) -> (error out=w1386:errorcluster)  [unwired: 1 in, 1 out]
      }
    }
  }
  n607 = control-ref of="PWR"() -> (w52:refnum<vi>)
  n608 = control-ref of="SM"() -> (w51:refnum<vi>)
  n609 = control-ref of="DC"() -> (w50:refnum<vi>)
  n610 = control-ref of="DM"() -> (w49:refnum<vi>)
  n611 = control-ref of="WS"() -> (w48:refnum<vi>)
  n612 = control-ref of="DS"() -> (w47:refnum<vi>)
  n613 = control-ref of="WC"() -> (w46:refnum<vi>)
  n614 = control-ref of="WA"() -> (w45:refnum<vi>)
  n615 = control-ref of="WM"() -> (w44:refnum<vi>)
  n616 = control-ref of="DA"() -> (w43:refnum<vi>)
  n617 = control-ref of="WH"() -> (w42:refnum<vi>)
  n618 = control-ref of="DH"() -> (w41:refnum<vi>)
  n619 = disable-structure "Conditional Disable Structure" shown="RUN_TIME_ENGINE==True&&OS==Win" {
    disable-tunnel: ["development" w1394 "Mac" "Linux"] -> w18
    frame condition #0 (active) {
    }
    frame condition #1 {
      n620 = Current VI's Path() -> (path=w1395:path)
      n621 = while {
        border: w1395 -> [_]
        tunnel: [w1396] -> w1394
        stop <- w1400 continue-if-true
        # "this VI only \nworks in Windows"
        n622 = feedback #1() -> (w1399:path)
        n623 = Strip Path(path=w1399) -> (stripped path=w1398:path)  [unwired: 1 out]
        n624 = feedback-in #1(w1398) -> ()
        n625 = File/Directory Info(path=w1398) -> (path out=w1397:path, error out=w1401:errorcluster)  [unwired: 1 in, 5 out]
        n626 = call <vilib>:"FileVersionInfo.vi"("error in (no error)"=w1401, "Application Path in"=w1397) -> ("error out"=w1400:errorcluster, "File Version Info"=w1396:string)  [unwired: 6 in, 2 out]
      }
    }
    frame condition #2 {
    }
    frame condition #3 {
    }
  }
  "version:" <- w18
  n627 = while {
    shift-right: [w1405] -> w40
    shift-left: w30 -> [w1410]
    tunnel: w38 -> [w1411]
    tunnel: w34 -> [w1408]
    tunnel: [w1407] -> w32
    tunnel: w17 -> [w1406]
    stop <- w1409 stop-if-true
    # "This loop is the producer loop."
    # "Event handler"
    n628 = event shown="[0] \"Start Button\": Value Change" {
      selector: w1408 -> [_ _ _ _ _ _]
      dyn-events: [_ _ _ _ _ _] -> w1407
      timeout: _ -> [_ _ _ _ _ _]
      tunnel: w1411 -> [w1417 w1442 w1446 w1449 w1460 _]
      tunnel: w1410 -> [_ _ w1448 _ w1455 w1461]
      tunnel: [w1416 w1443 w1447 _ w1458 w1461] -> w1405
      tunnel: [_ _ _ _ _ TRUE] -> w1404
      tunnel: w1406 -> [w1414 _ _ _ w1454 _]
      event "Start Button": Value Change {
        n629 = event-data() -> ("NewVal"=w1412:bool)  [unwired: 1 in, 5 out]
        n630 = case shown="False" w1412 {
          tunnel: w1417 -> [w1419 w1426]
          tunnel: [_ w1424] -> w1415
          tunnel: w1414 -> [_ w1422]
          tunnel: [w1420 w1421] -> w1413
          frame False {
            n631 = Enqueue Element(queue=w1419, element="idle") -> (error out=w1420:errorcluster)  [unwired: 2 in, 2 out]
          }
          frame True {
            n632 = case shown="\"AUTO\"" "Mode:" {
              selector: "Mode:" -> [w1429 w1438]
              tunnel: w1422 -> [w1431 w1434]
              tunnel: [w1427 w1435] -> w1421
              frame "AUTO" {
                n633 = Bundle("validate", "Mode"=w1429) -> (w1428:cluster{string, "Mode":T1})  [unwired: 1 in]
                n634 = Enqueue Element(queue=w1431, element=w1428) -> (error out=w1427:errorcluster)  [unwired: 2 in, 2 out]
              }
              frame "1 - PWR", Default {
                n635 = Enqueue Element(queue=w1434, element=cluster{"state":string, "element":T1} {"state"="clear screens", "element"=enum."AUTO"}) -> (queue out=w1433:refnum<queue>)  [unwired: 2 in, 2 out]
                n636 = Bundle("validate 4.9.12", "Mode"=w1438) -> (w1437:cluster{string, "Mode":T1})  [unwired: 1 in]
                n637 = Enqueue Element(queue=w1433, element=w1437) -> (error out=w1435:errorcluster)  [unwired: 2 in, 2 out]
              }
            }
            n638 = Enqueue Element(queue=w1426, element="running") -> (error out=w1424:errorcluster)  [unwired: 2 in, 2 out]
          }
        }
        n639 = Merge Errors(w1415, w1413) -> (w1416:errorcluster)
      }
      event "Options Button": Value Change {
        n640 = event-data() -> ("NewVal"=w1441:bool)  [unwired: 1 in, 5 out]
        n641 = Select(t="open paths" ("element"), s=w1441, f="close paths" ("element")) -> (s? t:f=w1439:string)
        n642 = Enqueue Element(queue=w1442, element=w1439) -> (error out=w1443:errorcluster)  [unwired: 2 in, 2 out]
      }
      event "Save Button": Value Change {
        n643 = event-data() -> ()  [unwired: 1 in, 6 out]
        n644 = Enqueue Element(queue=w1446, element="save config", error in (no error)=w1448) -> (error out=w1447:errorcluster)  [unwired: 1 in, 2 out]
      }
      event "Open part #": Value Change {
        n645 = event-data() -> ("NewVal"=w1450:bool)  [unwired: 1 in, 5 out]
        n646 = case shown="True" w1450 {
          tunnel: w1449 -> [_ w1452]
          frame False {
          }
          frame True {
            n647 = Enqueue Element(queue=w1452, element="get part" ("state")) -> ()  [unwired: 2 in, 3 out]
          }
        }
      }
      event Panel Close? {
        n648 = event-data() -> ()  [unwired: 1 in, 3 out]
        n649 = Enqueue Element At Opposite End(queue=w1454, element=cluster{"state":string, "element":T1} {"state"="kill loop", "element"=enum."AUTO"}, error in (no error)=w1455) -> (error out=w1456:errorcluster)  [unwired: 1 in, 2 out]
        n650 = Enqueue Element At Opposite End(queue=w1460, element="confirm quit" ("state"), error in (no error)=w1456) -> (error out=w1458:errorcluster)  [unwired: 1 in, 2 out]
        n651 = event-data("Discard?"=TRUE) -> ()  [unwired: 1 in, 1 out]
      }
      event User Event {
        n652 = event-data() -> ()  [unwired: 1 in, 3 out]
      }
    }
    n653 = Or(x=w1404, y=w1405) -> (x .or. y?=w1409:bool)
  }
  n654 = while {
    tunnel: w38 -> [w1473]
    shift-right: [w1468] -> _
    shift-left: w37 -> [w1469]
    tunnel: w35 -> [w1466]
    shift-right: [w1464] -> _
    shift-left: _ -> [w1465]
    tunnel: w17 -> [w1463]
    stop <- w1471 stop-if-true
    # "UI consummer"
    n655 = Dequeue Element(queue=w1473, error in (no error)=w1465) -> (queue out=w1467:refnum<queue>, element=w1470:string, error out=w1472:errorcluster)  [unwired: 1 in, 1 out]
    n656 = case shown="No Error" w1472 {
      selector: w1472 -> [w1476 _]
      tunnel: [_ TRUE] -> w1471
      tunnel: w1470 -> [w1475 _]
      tunnel: w1469 -> [w1481 _]
      tunnel: [w1480 _] -> w1468
      tunnel: w1467 -> [w1479 _]
      tunnel: w1466 -> [w1478 _]
      tunnel: [w1477 _] -> w1464
      tunnel: w1463 -> [w1474 _]
      frame No Error {
        n657 = case shown="\"read config\"" w1475 {
          tunnel: w1481 -> [w1495 w1507 w1513 w1524 w1537 w1547 w1554 w1563 w1574 w1582]
          tunnel: [w1494 w1507 w1513 w1524 w1537 w1547 w1554 w1563 w1574 w1582] -> w1480
          tunnel: w1479 -> [w1493 _ _ _ _ _ _ w1557 w1573 _]
          tunnel: w1478 -> [_ _ _ _ _ _ _ _ _ w1581]
          tunnel: [w1485 _ _ w1517 w1534 _ _ w1562 w1572 _] -> w1477
          tunnel: w1476 -> [_ _ _ _ _ _ _ _ _ _]
          tunnel: w1474 -> [_ _ _ w1516 _ _ _ _ _ _]
          frame "init", Default {
            n658 = Enqueue Element(queue=w1493, element="read config" ("state")) -> (queue out=w1491:refnum<queue>, error out=w1492:errorcluster)  [unwired: 2 in, 1 out]
            n659 = Enqueue Element(queue=w1491, element="idle" ("state"), error in (no error)=w1492) -> (error out=w1485:errorcluster)  [unwired: 1 in, 2 out]
            n660 = call "get part numbers.vi"() -> ("First part"=w1482:string)  [unwired: 10 in, 1 out]
            "Parte number" <- w1482
            n661 = Empty String/Path?(string/path=w1482) -> (empty?=w1483:bool)
            n662 = case shown="False" w1483 {
              tunnel: [w1497 _] -> w1484
              tunnel: w1482 -> [w1496 _]
              frame False {
                n663 = Concatenate Strings(w1496, ".ini" ("string")) -> (w1497:string)
              }
              frame True {
              }
            }
            n664 = control-ref of="footer splitter"() -> (w1486:refnum<vi>)
            n665 = control-ref of="Path: 4.9.12.XXXX"() -> (w1490:refnum<vi>)
            n666 = control-ref of="Path: Mi app"() -> (w1489:refnum<vi>)
            n667 = Bundle By Name(cluster=w1495, "Path: Version"=w1490, "Path: My app"=w1489, "footer splitter"=w1486, "Part number (.ini)"=w1484) -> (w1494:T4)
          }
          frame "idle" {
            n668 = property on="Open part #" class="Bool (strict)"("DisabledEnum"=T2."Enabled" ("Disabled"), "Value"=FALSE ("Open part #")) -> ()  [unwired: 2 in, 2 out]
            n669 = property on="Start Button" class="Bool (strict)"("Value"=FALSE ("Save button"), "DisabledEnum"=T2."Enabled" ("Disabled")) -> ()  [unwired: 2 in, 2 out]
            n670 = property on="Options Button" class="Bool (strict)"("Val(Sgnl)"=FALSE ("Options Button"), "DisabledEnum"=T2."Enabled" ("Disabled")) -> ()  [unwired: 2 in, 2 out]
            n671 = property on="Save Button" class="Bool (strict)"("Value"=FALSE ("Save button"), "DisabledEnum"=T2."Enabled" ("Disabled")) -> ()  [unwired: 2 in, 2 out]
          }
          frame "running" {
            n672 = property on="Options Button" class="Bool (strict)"("Val(Sgnl)"=FALSE ("Value (Signaling)")) -> ()  [unwired: 2 in, 2 out]
            n673 = property on="Start Button" class="Bool (strict)"("DisabledEnum"=T2."Disabled and Grayed Out" ("Disabled")) -> ()  [unwired: 2 in, 2 out]
            n674 = property on="Tab Control" class="TabCtl (strict)"("Value"=enum32{"Micros", "Micro", "SSH"}."Micros" ("Tab Control"), "DisabledEnum"=T2."Disabled" ("Disabled")) -> ()  [unwired: 2 in, 2 out]
            n675 = property on="Open part #" class="Bool (strict)"("DisabledEnum"=T2."Disabled and Grayed Out" ("Disabled")) -> ()  [unwired: 2 in, 2 out]
          }
          frame "read config" {
            n676 = Unbundle By Name(w1524) -> ("Path: Version"=w1522:refnum<vi>, "Path: My app"=w1523:refnum<vi>, "Part number (.ini)"=w1514:string)
            n677 = call "config handler.vi"("Operation"=enum16{"Open", "Write", "Read", "Close"}."Open", "Part number (.ini)"=w1514) -> ("Error Out"=w1527:errorcluster)  [unwired: 8 in, 1 out]
            n678 = call "config handler.vi"("Operation"=enum16{"Open", "Write", "Read", "Close"}."Read", "error in (no error)"=w1527) -> ("Read values"=w1521:T9)  [unwired: 8 in, 1 out]
            n679 = Unbundle By Name(w1521) -> ("Path: 4.9.12.XXXX"=w1520:path, "Path: Mi app"=w1519:path)
            n680 = property class="Path"(reference=w1522, "Value"=w1520) -> ()  [unwired: 1 in, 2 out]
            n681 = property class="Path"(reference=w1523, "Value"=w1519) -> (error out=w1518:errorcluster)  [unwired: 1 in, 1 out]
            n682 = Enqueue Element(queue=w1516, element=cluster{"state":string, "element":T1} {"state"="init", "element"=enum."AUTO"}, error in (no error)=w1518) -> (error out=w1517:errorcluster)  [unwired: 1 in, 2 out]
          }
          frame "save config" {
            n683 = Bundle By Name(cluster=T9 {"Path: 4.9.12.XXXX"=path "", "Path: Mi app"=path "", "Username"="", "Password"=""} ("Write values"), "Path: 4.9.12.XXXX"="Path: 4.9.12.XXXX", "Path: Mi app"="Path: Mi app") -> (w1531:T9)
            n684 = call "config handler.vi"("Operation"=enum16{"Open", "Write", "Read", "Close"}."Write", "Write values"=w1531) -> ("Error Out"=w1533:errorcluster)  [unwired: 8 in, 1 out]
            n685 = case shown="No Error" w1533 {
              selector: w1533 -> [w1540 w1541]
              tunnel: [w1540 w1541] -> w1535
              frame No Error {
                n686 = call "Custom Message.vi"("Boolean Text"="OK", "MSG"="\n\n¡Se ha guardado con éxito!") -> ()  [unwired: 10 in]
              }
              frame Error {
              }
            }
            n687 = property on="Save Button" class="Bool (strict)"(error in=w1535, "Value"=FALSE ("Save button")) -> (error out=w1534:errorcluster)  [unwired: 1 in, 1 out]
          }
          frame "open paths" {
            n688 = control-ref of="This VI"() -> (w1546:refnum<vi>)
            n689 = property class="VI"(reference=w1546) -> ("Panel"=w1545:refnum<vi>)  [unwired: 1 in, 2 out]
            n690 = property class="Pnl"(reference=w1545) -> ("Height"=w1544:u32)  [unwired: 1 in, 2 out]
            n691 = Unbundle By Name(w1547) -> ("footer splitter"=w1548:refnum<vi>)
            n692 = Subtract(x=w1544, y=u32 125) -> (x-y=w1542:u32)
            n693 = property class="Splitter"(reference=w1548, "Position"=w1542) -> ()  [unwired: 1 in, 2 out]
          }
          frame "close paths" {
            n694 = control-ref of="This VI"() -> (w1553:refnum<vi>)
            n695 = property class="VI"(reference=w1553) -> ("Panel"=w1552:refnum<vi>)  [unwired: 1 in, 2 out]
            n696 = property class="Pnl"(reference=w1552) -> ("Height"=w1551:u32)  [unwired: 1 in, 2 out]
            n697 = Unbundle By Name(w1554) -> ("footer splitter"=w1555:refnum<vi>)
            n698 = Subtract(x=w1551, y=u32 28) -> (x-y=w1550:u32)
            n699 = property class="Splitter"(reference=w1555, "Position"=w1550) -> ()  [unwired: 1 in, 2 out]
          }
          frame "get part" {
            n700 = Enqueue Element(queue=w1557, element="read config") -> ()  [unwired: 2 in, 3 out]
            n701 = property on="Open part #" class="Bool (strict)"("Value"=FALSE ("Open part #")) -> (error out=w1559:errorcluster)  [unwired: 2 in, 1 out]
            n702 = call "Available parts Display.vi"("error in"=w1559) -> ("Cancel?"=w1561:bool, "Part Number"=w1558:string, "error out"=w1562:errorcluster)  [unwired: 11 in, 1 out]
            n703 = case shown="False" w1561 {
              tunnel: w1558 -> [w1566 _]
              frame False {
                n704 = control-ref of="Parte number"() -> (w1567:refnum<vi>)
                n705 = property class="Str"(reference=w1567, "Value"=w1566) -> (error out=w1564:errorcluster)  [unwired: 1 in, 1 out]
                n706 = call "config handler.vi"("Operation"=enum16{"Open", "Write", "Read", "Close"}."Close", "error in (no error)"=w1564) -> ()  [unwired: 8 in, 2 out]
              }
              frame True {
              }
            }
          }
          frame "confirm quit" {
            n707 = call "Custom two options Message.vi"("MSG"="\n\n¿Seguro que quiere cerrar\nla aplicación?" ("message"), "Red text"="Cancelar" ("F button name (\"Cancel\")"), "Green text"="Si" ("T button name (\"OK\")")) -> ("Ok?"=w1568:bool)  [unwired: 8 in]
            n708 = case shown="True" w1568 {
              tunnel: w1573 -> [_ w1577]
              tunnel: [_ w1575] -> w1572
              frame False {
              }
              frame True {
                n709 = Enqueue Element At Opposite End(queue=w1577, element="exit" ("state")) -> (error out=w1575:errorcluster)  [unwired: 2 in, 2 out]
              }
            }
          }
          frame "exit" {
            n710 = call "config handler.vi"("Operation"=enum16{"Open", "Write", "Read", "Close"}."Close") -> ("Error Out"=w1580:errorcluster)  [unwired: 9 in, 1 out]
            n711 = Generate User Event(user event=w1581, event data cluster="stop app" ("event data"), error in=w1580) -> ()  [unwired: 1 in, 2 out]
          }
        }
      }
      frame Error {
        # "Return true in any case that should stop the loop."
        n712 = disable-structure "Conditional Disable Structure" shown="RUN_TIME_ENGINE==True&&OS==Win" {
          frame condition #0 (active) {
          }
          frame condition #1 {
            n713 = Quit LabVIEW(quit? (T)=TRUE) -> ()
          }
        }
      }
    }
  }
  n714 = Build Array(w52, w51, w50, w49, w48, w47, w46, w45, w44, w43, w42, w41) -> (w53:refnum<vi>[])
  n715 = for {
    tunnel: w53 -> [w1585] mode=indexing
    n716 = property class="Bool (strict)"(reference=w1585, "DisabledEnum"=T2."Disabled" ("Disabled")) -> ()  [unwired: 1 in, 2 out]
  }
  n717 = Release Queue(queue=w38, error in (no error)=w40) -> (error out=w33:errorcluster)  [unwired: 1 in, 2 out]
  n718 = Unregister For Events(event registration refnum=w32, error in=w33) -> (error out=w29:errorcluster)
  n719 = Release Queue(queue=w17, error in (no error)=w29) -> ()  [unwired: 1 in, 3 out]
  "Status" <- ""
